vi "fast scanner v1.1.vi"() -> ()   [LabVIEW 2015]
uses:
  outofrange.ctl
  loopclock.ctl
  libs/fast scanner.ctl
  <vilib>/Utility/file.llb/Write Delimited Spreadsheet (I64).vi
  Zaber A Series/Zaber A Series.lvlib
panel:
  in  "Data folder path":path=path "d:/Users/XRF/Desktop/Scan DATA"
  out "DANTE loaded":bool
  out "IP added":bool
  out "Library Initialized":bool
  out "DANTE configured":bool
  out "Enum":T1=enum."MoveToStartPoint"
  out "scan mode":bool
  out "Port":refnum<visa-resource-name>
  out "MotorsReady":bool
  out "Speed 2":T2 scale=0.0..30.0
  in  "Tab Control":T3(tab)
  in  "StopMotion":bool
  in  "GoToZ":bool
  in  "GoToY":bool
  in  "GoToX":bool
  in  "GoTo Z [mm]":dbl format="%#.8g"
  in  "GoTo Y [mm]":dbl format="%#.8g"
  in  "GoTo X [mm]":dbl format="%#.8g"
  in  "Reduced Speed":bool
  in  "Speed Z [mm/s]":dbl(slide) caption="Z Speed\n[mm/s]" min=0.5 max=10.0 step=0.5 scale=0.5..10.0
  in  "XY Speed\n[mm/s]":dbl(slide)=1.0 min=1.0 max=75.0 step=1.0 scale=1.0..75.0
  in  "Away":bool
  in  "Closer":bool
  in  "Right":bool
  in  "Left":bool
  in  "Down":bool
  in  "Up":bool
  out "X [mm]":dbl format="%#.8g"
  out "Y [mm]":dbl format="%#.8g"
  out "Z [mm]":dbl format="%#.3g"
  out "Assignment":cluster{"Microstep Size":dbl, "Device":string}[](array[cluster])
  in  "Acceleration [mm/s^2]":dbl=1.0 min=1.0 max=488.0
  out "SpectraPlot":dbl[](graph) caption="Waveform Graph"
  in  "APPEARANCE_CursorVis":bool
  in  "APPEARANCE_Log/Lin":bool=TRUE
  out "stats out":T4
  out "identifier out":string
  in  "IP Address":string="10.96.0.110"
  out "Progress":u32 caption="%" min=1 step=1
  in  "Preset Time [s]":dbl=1.0 min=0.2 step=0.1
  out "Elapsed Time":dbl caption="Elapsed Time [s]" format="%#_4g"
  in  "MEASUREMENT_Start":bool
  in  "INIT DANTE":bool
  in  "Close DANTE":bool
  out "ROI Begin":u32 caption="ROI begin channel"
  out "ROI End":u32 caption="ROI end channel"
  in  "X velocity [mm/s]":dbl=50.0 min=0.0 step=0.1
  out "Total scan time [s]":dbl=1.0 min=0.0 step=0.1
  out "Total line time [s]":dbl=1.0 min=0.0 step=0.1
  out "Acq time [s]":dbl=1.0 min=0.0 step=0.1
  in  "AcqStartDelay":dbl caption="Acq start delay [ms]"
  in  "Abort scan":bool
  out "Acc time [s]":dbl=1.0 min=0.0 step=0.1
  out "Acc dist [mm]":dbl=1.0 caption="Single line measurement time:" min=0.0 step=0.1
  in  "X accel":dbl caption="X acceleration [mm/s^2]"
  out "Line #":i32=1 caption="/" min=0 step=1
  out "X scan velocity [mm/s]":dbl=1.0 min=0.0 step=0.1
  in  "QUICKSCAN_Start":bool
  out "Y error":T5
  out "X error":T5
  out "total # of points":i32=1 min=0 step=1
  out "Y steps":i32=1 min=1 step=1
  out "X steps":i32=1 min=1 step=1
  in  "step Y [mm]":dbl=1.0 min=0.0 step=0.1
  in  "Y end [mm]":dbl=1.0
  in  "Y start [mm]":dbl
  in  "step X [mm]":dbl=1.0 min=0.0 step=0.1
  in  "X end [mm]":dbl=1.0
  in  "X start [mm]":dbl
  in  "PresetVal":u32 caption="Time per pixel [ms]"
  out "X speed error":T5
  out "total line #":i32=1 caption="/" min=0 step=1
  out "Return movement time [s]":dbl=1.0 min=0.0 step=0.1
  out "ROI map":u32[][](graph)
  out "Sum spectra":u32[](graph)
  out "Spectra":u16[][](graph)
  out "scan timing [ms]":dbl[][](array[numeric])
  out "Y positions array":dbl[](array[numeric])
  out "X start position":dbl
  out "X end position":dbl
  in  "Precision [mm]":dbl=0.1
  out "ZaberError":errorcluster
  out "Loop Speed [1/s]":dbl caption="Elapsed Time [s]" format="%#_2f"
  # "waiting \ntill stage \nreaches \nproper speed"
  # "sending \nmovement \ncommand"
  # "waiting till \nstage stops \n(breaking)"
  # "aquisition"
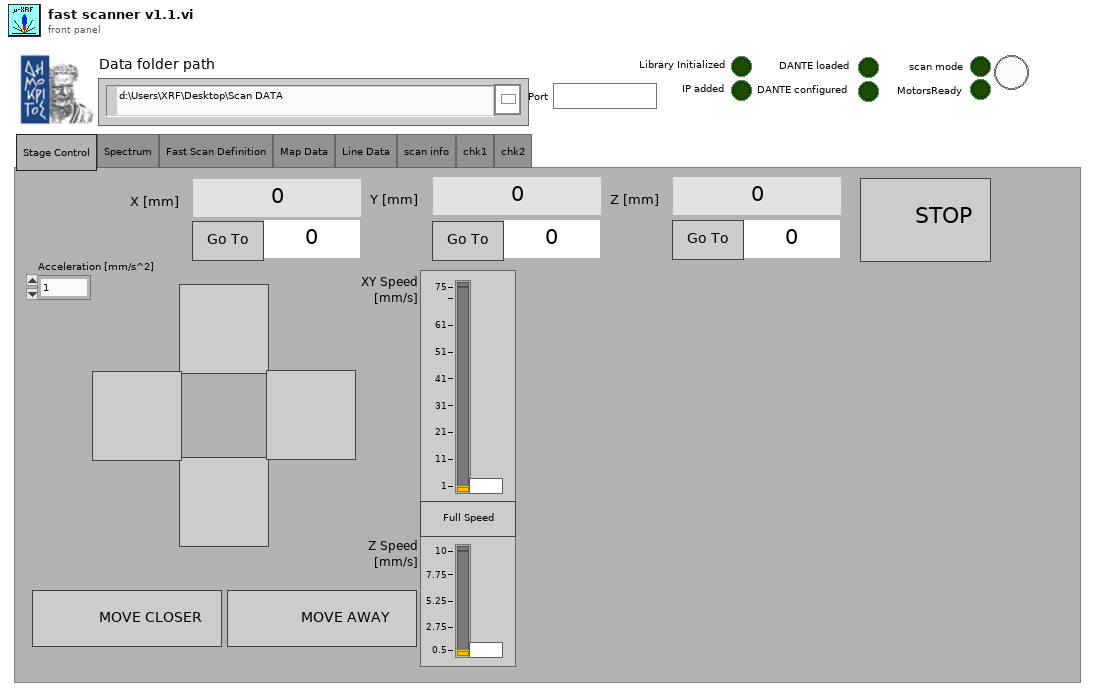
[diagram p1: front panel]
types:
  T1 = typedef "fast scanner.ctl" = enum16{"Initialisation", "IDLE", "Acquire", "PrepareMap", "MoveToStartPoint", "AcquireLine", "Close"}
  T2 = typedef "loopclock.ctl" = dbl
  T3 = enum32{"Stage Control", "Spectrum", "Fast Scan Definition", "Map Data", "Line Data", "scan info", "chk1", "chk2"}
  T4 = cluster{u64, u64, dbl, dbl, u32, u32, u32, u32, u32, u32, u32, u32, u32, u32, u32}
  T5 = typedef "outofrange.ctl" = bool
  T6 = cluster{"X min":dbl, "X max":dbl, "Y min":dbl, "Y max":dbl, "Z min":dbl, "Z max":dbl}
  T7 = enum32{"Size Tabs To Contents", "Size All Tabs to Largest Tab", "Fixed Tab Size"}
  T8 = enum8{"Enabled", "Disabled", "Disabled and Grayed Out"}
  T9 = typedef "LVMinMaxIncTypeDef.ctl" = cluster{"Minimum":dbl, "Maximum":dbl, "Increment":dbl}
  T10 = typedef "LVRangeTypeDef.ctl" = cluster{"Minimum":dbl, "Maximum":dbl, "Increment":dbl, "Minor Increment":dbl, "Start":dbl}
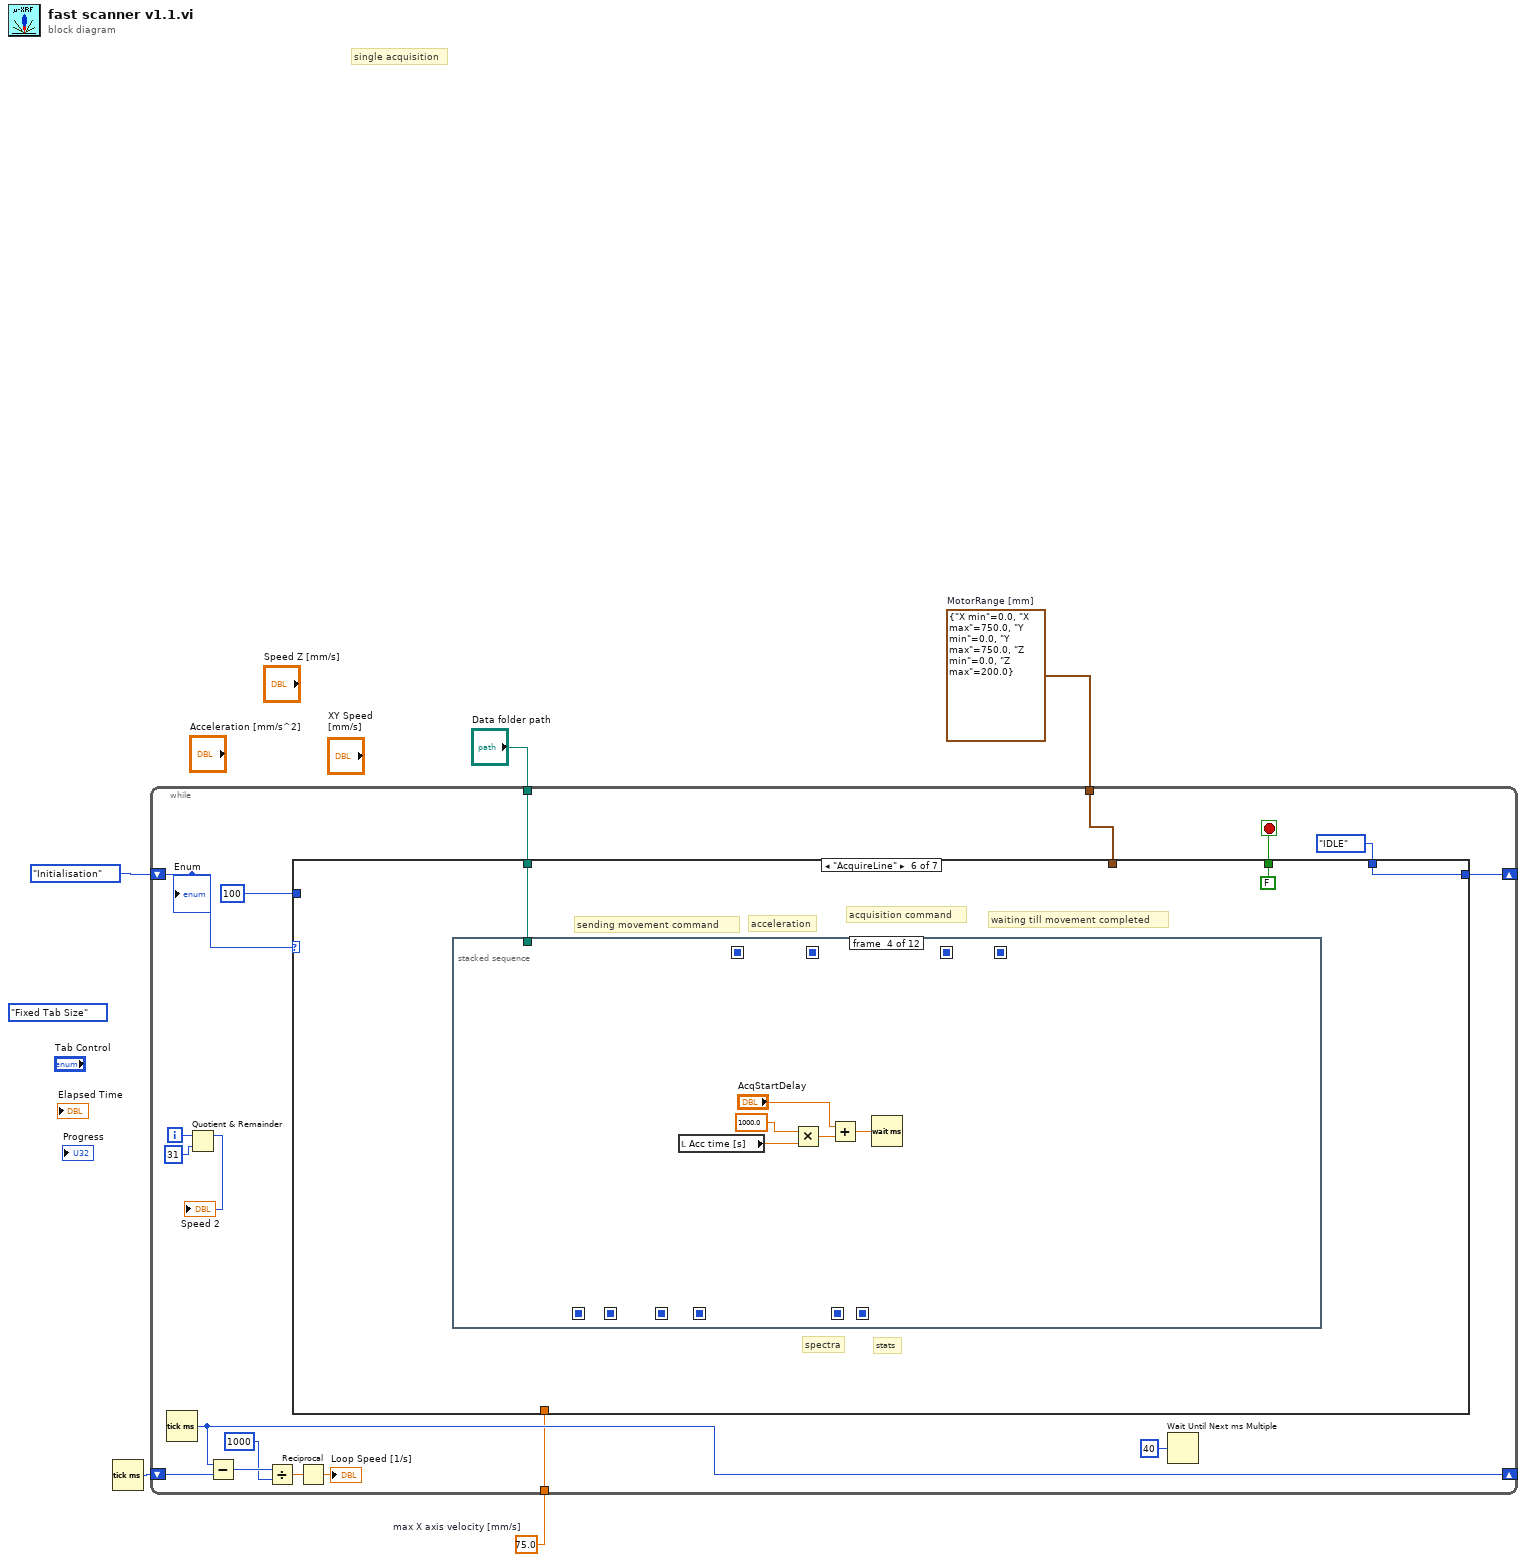
[diagram p0: block diagram]
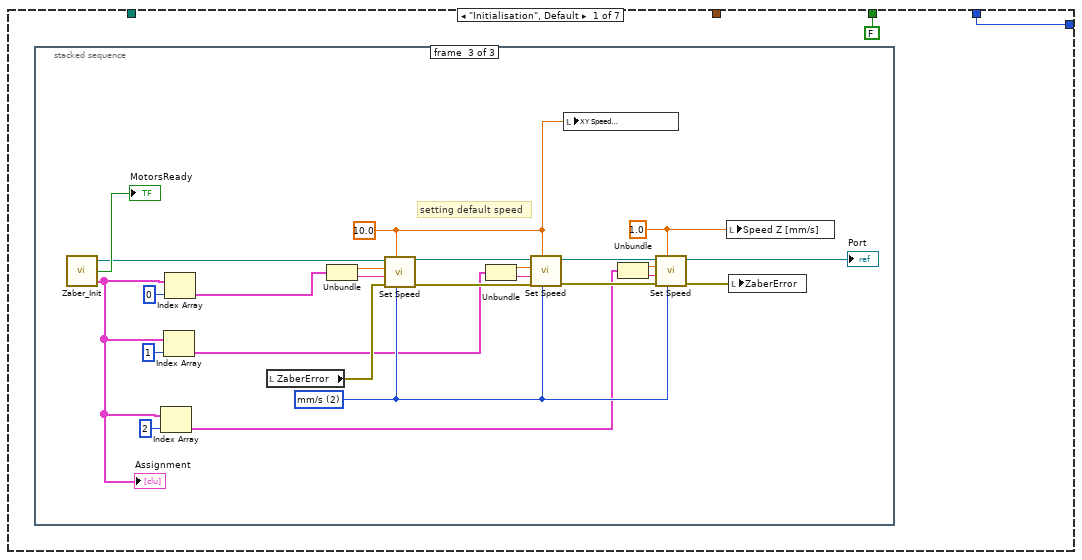
[diagram p2: hidden frame]
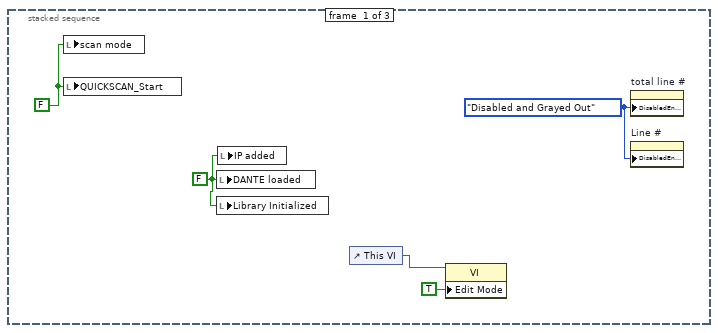
[diagram p3: hidden frame]
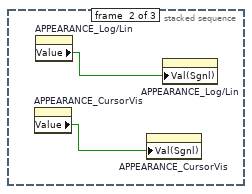
[diagram p4: hidden frame]
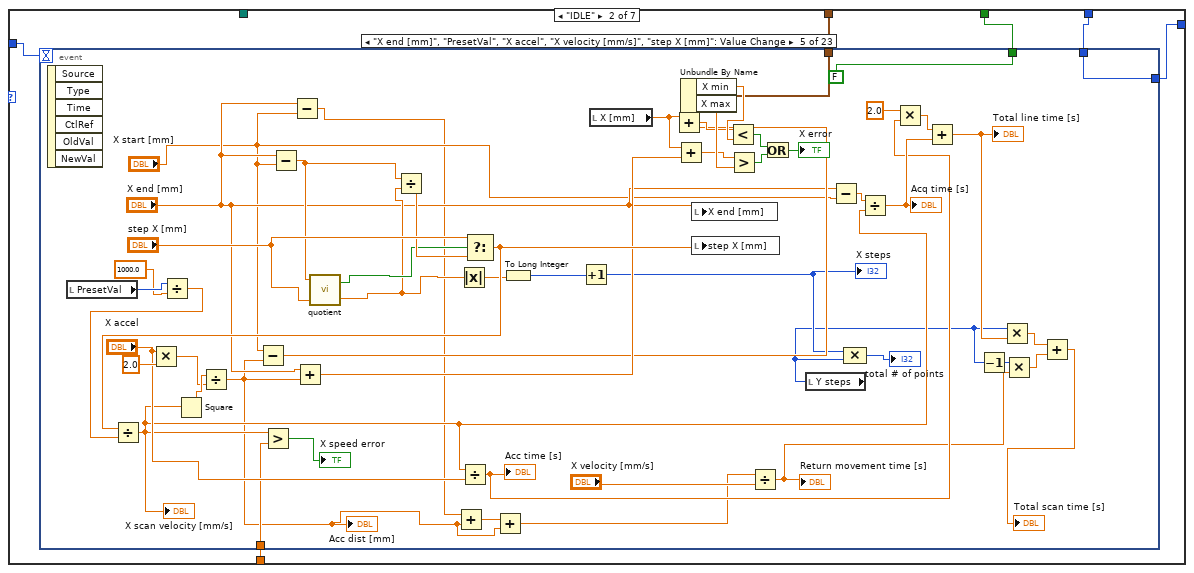
[diagram p5: hidden frame]
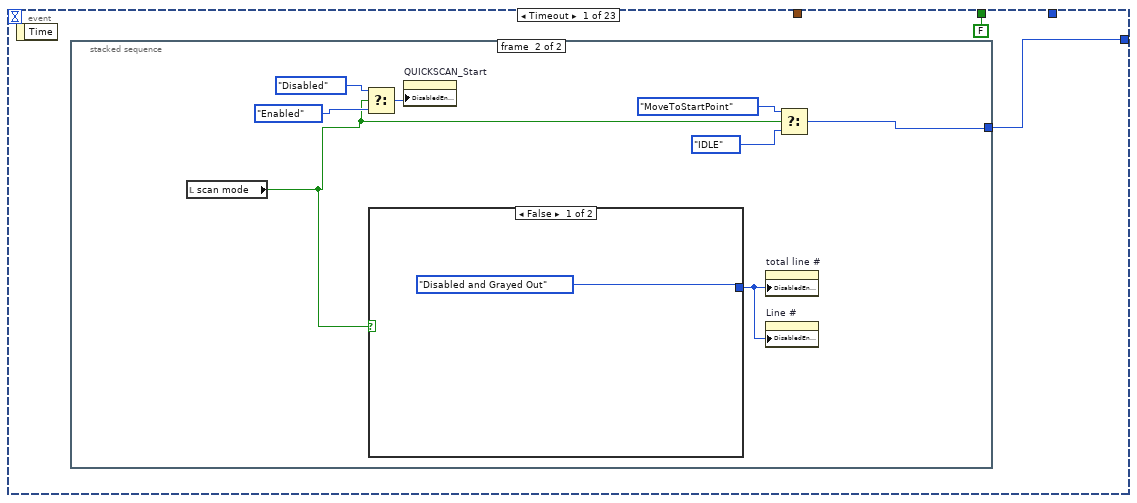
[diagram p6: hidden frame]
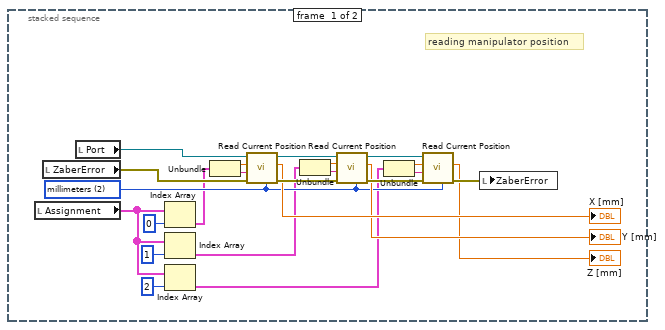
[diagram p7: hidden frame]
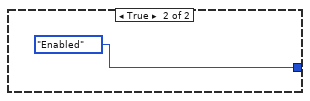
[diagram p8: hidden frame]
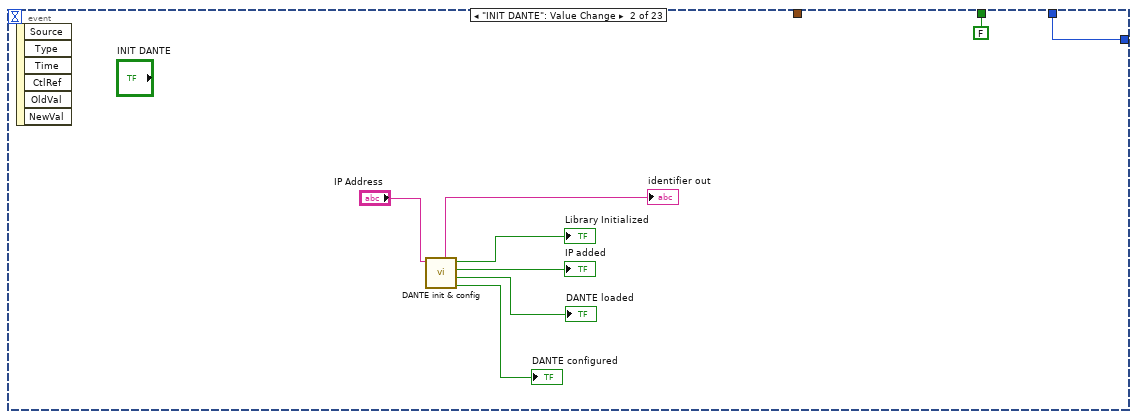
[diagram p9: hidden frame]
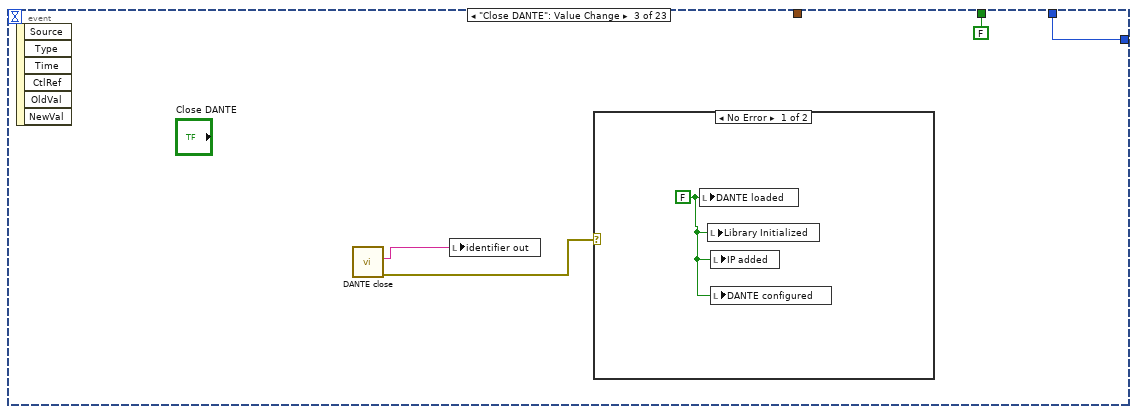
[diagram p10: hidden frame]
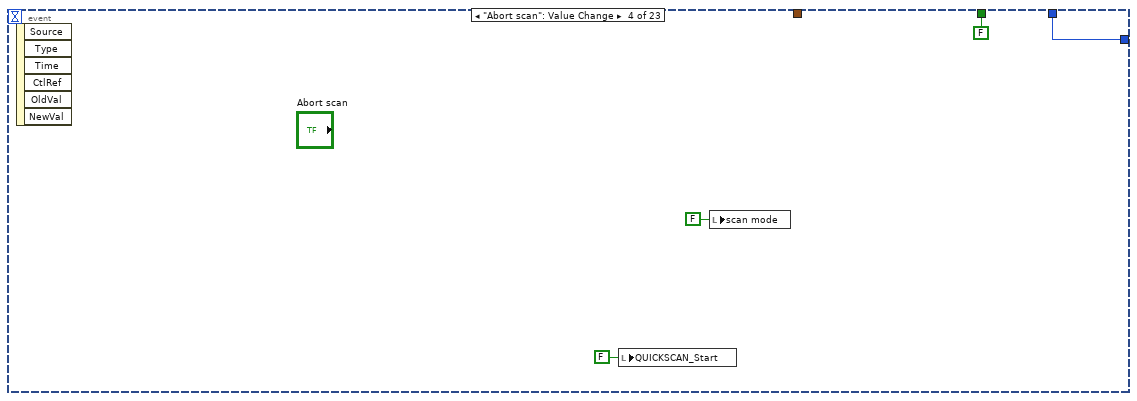
[diagram p12: hidden frame]
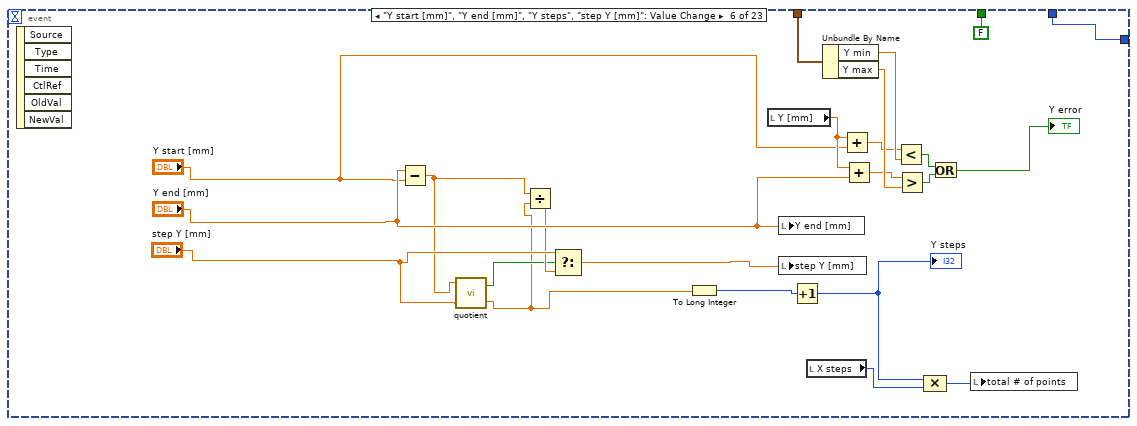
[diagram p13: hidden frame]
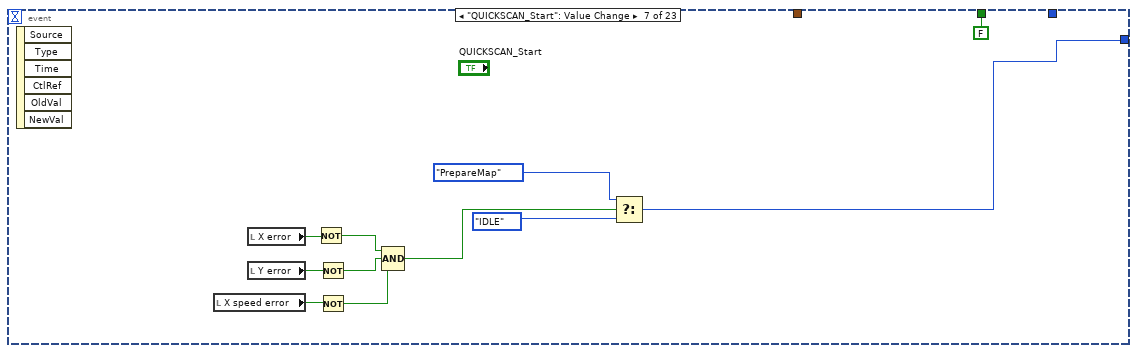
[diagram p14: hidden frame]
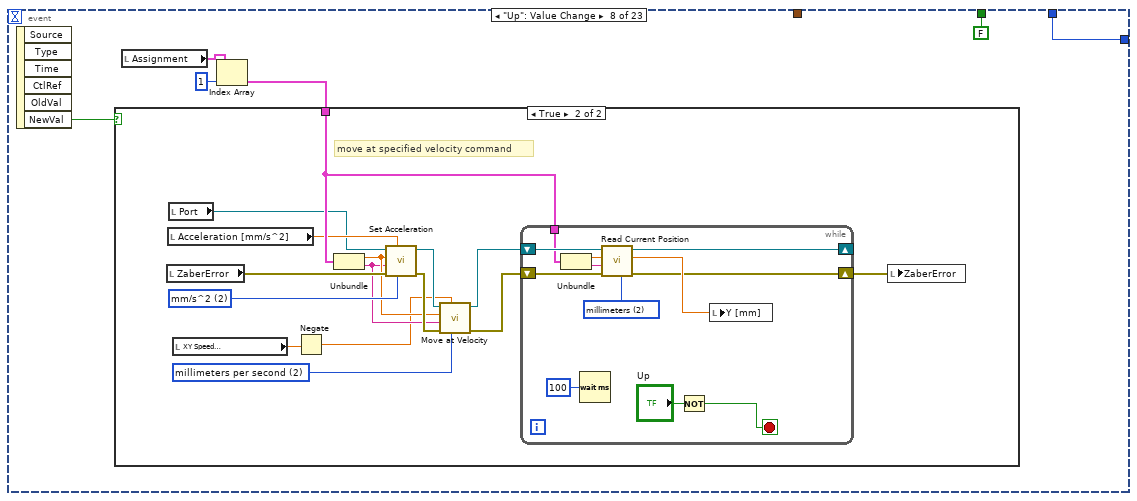
[diagram p15: hidden frame]
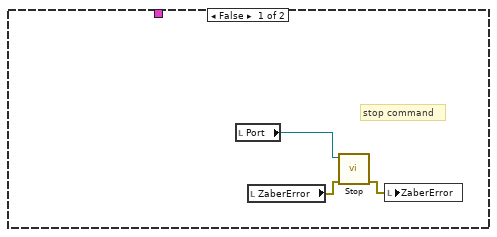
[diagram p16: hidden frame]
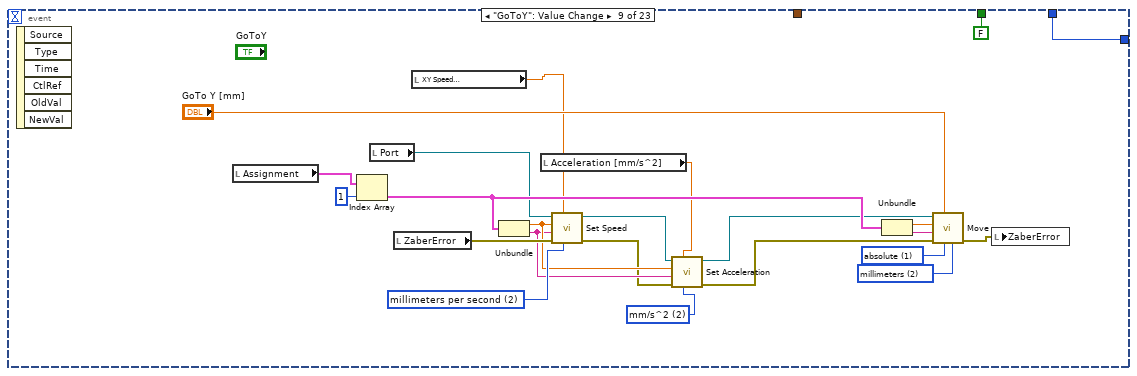
[diagram p17: hidden frame]
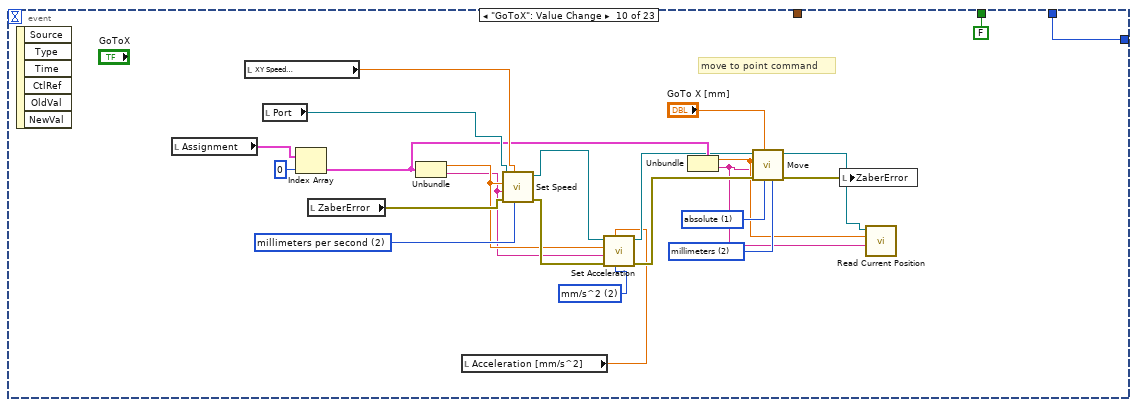
[diagram p18: hidden frame]
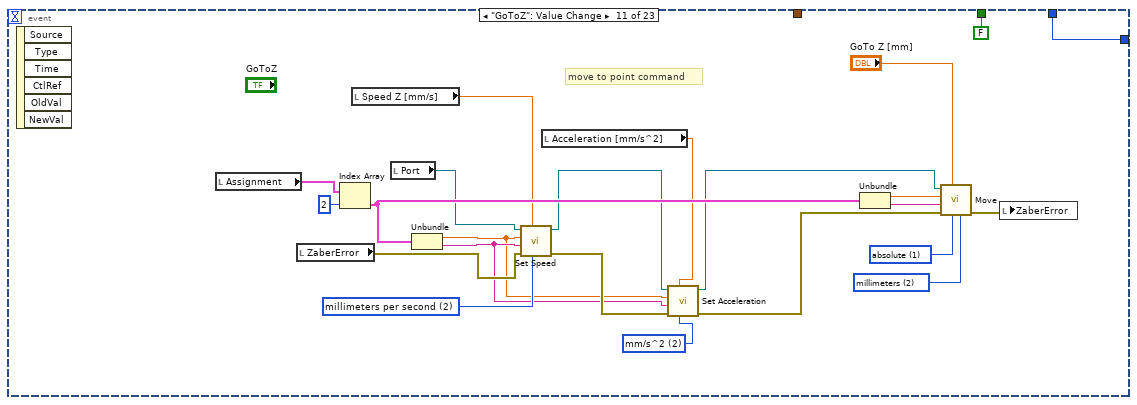
[diagram p19: hidden frame]
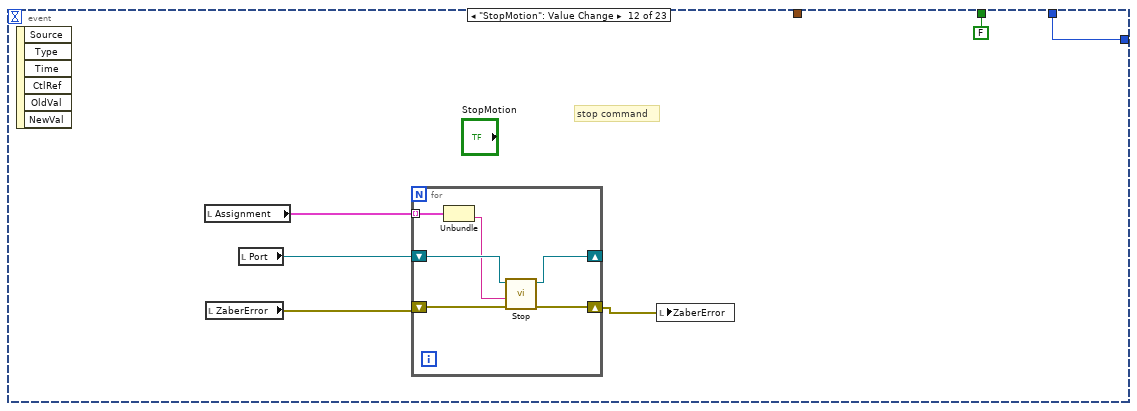
[diagram p20: hidden frame]
diagram:
  w2 = 75.0  # max X axis velocity [mm/s]
  w4 = T6 {"X min"=0.0, "X max"=750.0, "Y min"=0.0, "Y max"=750.0, "Z min"=0.0, "Z max"=200.0}  # MotorRange [mm]
  (unwired) T7."Fixed Tab Size" ("Tab Size")
  # "single acquisition"
  n1 = Tick Count (ms)() -> (millisecond timer value=w5:u32)
  n2 = while {
    shift-right: [w12] -> _
    shift-left: fast_scanner."Initialisation" ("Enum") -> [w8]
    shift-right: [w19] -> _
    shift-left: w5 -> [w23]
    tunnel: w4 -> [w9]
    tunnel: w2 -> [w7]
    tunnel: "Data folder path" -> [w6]
    i -> [w18]
    stop <- w11 stop-if-true
    n3 = Tick Count (ms)() -> (millisecond timer value=w19:u32)
    n4 = Quotient & Remainder(x=w18, y=31) -> (x-y*floor(x/y)=→"Speed 2":i32)  [unwired: 1 out]
    n5 = Subtract(x=w19, y=w23) -> (x-y=w21:u32)
    n6 = Divide(x=w21, y=u32 1000) -> (x/y=w22:dbl)
    n7 = case shown="\"AcquireLine\"" w8 {
      tunnel: 100 ("LoopTimer [ms]") -> [_ w59 _ _ _ _ _]
      tunnel: [w25 w61 fast_scanner."IDLE" ("Enum") w573 fast_scanner."AcquireLine" ("Enum") w683 fast_scanner."Close" ("Enum")] -> w12
      tunnel: [FALSE ("VI stop") w60 FALSE ("VI stop") FALSE ("VI stop") FALSE ("VI stop") FALSE ("VI stop") TRUE ("VI stop")] -> w11
      tunnel: fast_scanner."IDLE" ("Enum") -> [w25 w63 _ w573 _ w683 _]
      tunnel: w9 -> [_ w62 _ _ _ _ _]
      tunnel: w7 -> [_ w58 _ _ _ _ _]
      tunnel: w6 -> [_ _ _ _ _ w682 _]
      frame "Initialisation", Default {
        n8 = stacked-sequence {
          frame #0 {
            w26 = FALSE ("DANTE loaded")
            w27 = T8."Disabled and Grayed Out" ("Disabled")
            w28 = FALSE ("batch mode")
            n9 = local write "scan mode"(w28) -> ()
            n10 = local write "QUICKSCAN_Start"(w28) -> ()
            n11 = local write "DANTE loaded"(w26) -> ()
            n12 = local write "Library Initialized"(w26) -> ()
            n13 = local write "IP added"(w26) -> ()
            n14 = control-ref of="This VI"() -> (w29:refnum<vi>)
            n15 = property class="VI"(reference=w29, "Edit Mode"=TRUE ("Edit Mode On Open")) -> ()  [unwired: 1 in, 2 out]
            n16 = property on="total line #" class="DigNum (strict)"("DisabledEnum"=w27) -> ()  [unwired: 2 in, 2 out]
            n17 = property on="Line #" class="DigNum (strict)"("DisabledEnum"=w27) -> ()  [unwired: 2 in, 2 out]
          }
          frame #1 {
            n18 = property on="APPEARANCE_CursorVis" class="Bool (strict)"() -> ("Value"=w31:bool)  [unwired: 2 in, 2 out]
            n19 = property on="APPEARANCE_Log/Lin" class="Bool (strict)"() -> ("Value"=w32:bool)  [unwired: 2 in, 2 out]
            n20 = property on="APPEARANCE_CursorVis" class="Bool (strict)"("Val(Sgnl)"=w31) -> ()  [unwired: 2 in, 2 out]
            n21 = property on="APPEARANCE_Log/Lin" class="Bool (strict)"("Val(Sgnl)"=w32) -> ()  [unwired: 2 in, 2 out]
          }
          frame #2 {
            w42 = 1.0 ("New Speed")
            w43 = 10.0 ("New Speed")
            w46 = u16 2 items=["device units", "microns/s", "mm/s", "inches/s", "degrees/s"] ("Units (0: data)")
            # "setting default speed"
            n22 = call "Zaber_Init.vi"() -> ("Assignment"=w47:cluster{"Microstep Size":dbl, "Device":string}[], "Axes Ass"=→"MotorsReady":bool, "VISA resource name out"=w55:refnum<visa-resource-name>)
            "Assignment" <- w47
            n23 = Index Array(array=w47, index=2) -> (element=w34:cluster{"Microstep Size":dbl, "Device":string})
            n24 = Index Array(array=w47, index=1) -> (element=w36:cluster{"Microstep Size":dbl, "Device":string})
            n25 = Index Array(array=w47, index=0) -> (element=w41:cluster{"Microstep Size":dbl, "Device":string})
            n26 = local read "ZaberError"() -> (w56:errorcluster)
            n27 = Unbundle(w41) -> ("Microstep Size"=w40:dbl, "Device"=w39:string)
            n28 = call "Set Speed.vi"("Units (0: data)"=w46, "New Speed"=w43, "error in (no error)"=w56, "Device and Axis"=w39, "Microstep Size (0)"=w40, "VISA resource name"=w55) -> ("error out"=w52:errorcluster, "VISA resource name out"=w51:refnum<visa-resource-name>)  [unwired: 4 in]
            n29 = Unbundle(w36) -> ("Microstep Size"=w37:dbl, "Device"=w38:string)
            n30 = call "Set Speed.vi"("Units (0: data)"=w46, "New Speed"=w43, "error in (no error)"=w52, "Device and Axis"=w38, "Microstep Size (0)"=w37, "VISA resource name"=w51) -> ("error out"=w49:errorcluster, "VISA resource name out"=w50:refnum<visa-resource-name>)  [unwired: 4 in]
            n31 = local write "XY Speed\n[mm/s]"(w43) -> ()
            n32 = Unbundle(w34) -> ("Microstep Size"=w35:dbl, "Device"=w33:string)
            n33 = call "Set Speed.vi"("Units (0: data)"=w46, "New Speed"=w42, "error in (no error)"=w49, "Device and Axis"=w33, "Microstep Size (0)"=w35, "VISA resource name"=w50) -> ("error out"=w45:errorcluster, "VISA resource name out"=→"Port":refnum<visa-resource-name>)  [unwired: 4 in]
            n34 = local write "Speed Z [mm/s]"(w42) -> ()
            n35 = local write "ZaberError"(w45) -> ()
          }
        }
      }
      frame "IDLE" {
        n36 = event shown="[4] \"X end [mm]\", \"PresetVal\", \"X accel\", \"X velocity [mm/s]\", \"step X [mm]\": Value Change" {
          selector: _ -> [_ _ _ _ _ _ _ _ _ _ _ _ _ _ _ _ _ _ _ _ _ _ _]
          dyn-events: _ -> [_ _ _ _ _ _ _ _ _ _ _ _ _ _ _ _ _ _ _ _ _ _ _]
          timeout: w59 -> [_ _ _ _ _ _ _ _ _ _ _ _ _ _ _ _ _ _ _ _ _ _ _]
          tunnel: [FALSE ("VI stop") FALSE ("VI stop") FALSE ("VI stop") FALSE ("VI stop") FALSE ("VI stop") FALSE ("VI stop") FALSE ("VI stop") FALSE ("VI stop") FALSE ("VI stop") FALSE ("VI stop") FALSE ("VI stop") FALSE ("VI stop") FALSE ("VI stop") FALSE ("VI stop") FALSE ("VI stop") FALSE ("VI stop") FALSE ("VI stop") FALSE ("VI stop") TRUE ("VI stop") FALSE ("VI stop") FALSE ("VI stop") FALSE ("VI stop") FALSE ("VI stop")] -> w60
          tunnel: [w64 w107 w111 w115 w168 w189 w192 w206 w260 w284 w307 w314 w325 w360 w395 w431 w466 w510 w527 fast_scanner."Acquire" ("Enum") w545 w550 w554] -> w61
          tunnel: w63 -> [_ w107 w111 w115 w168 w189 _ w206 w260 w284 w307 w314 w325 w360 w395 w431 w466 w510 _ _ w545 w550 w554]
          tunnel: w62 -> [_ _ _ _ w156 w175 _ _ _ _ _ _ _ _ _ _ _ _ _ _ _ _ _]
          tunnel: w58 -> [_ _ _ _ w145 _ _ _ _ _ _ _ _ _ _ _ _ _ _ _ _ _ _]
          event Timeout {
            n37 = event-data() -> ()  [unwired: 1 in, 1 out]
            n38 = stacked-sequence {
              tunnel: [_ w97] -> w64
              frame #0 {
                w76 = u16 2 items=["microsteps", "microns", "millimeters", "inches"] ("Units (0: microsteps)")
                # "reading manipulator position"
                n39 = local read "Assignment"() -> (w75:cluster{"Microstep Size":dbl, "Device":string}[])
                n40 = local read "ZaberError"() -> (w88:errorcluster)
                n41 = local read "Port"() -> (w89:refnum<visa-resource-name>)
                n42 = Index Array(array=w75, index=0) -> (element=w74:cluster{"Microstep Size":dbl, "Device":string})
                n43 = Index Array(array=w75, index=1) -> (element=w70:cluster{"Microstep Size":dbl, "Device":string})
                n44 = Index Array(array=w75, index=2) -> (element=w66:cluster{"Microstep Size":dbl, "Device":string})
                n45 = Unbundle(w74) -> ("Microstep Size"=w73:dbl, "Device"=w72:string)
                n46 = call "Read Current Position.vi"("Units (0: microsteps)"=w76, "error in (no error)"=w88, "Device and Axis"=w72, "Microstep Size (0)"=w73, "VISA resource name"=w89) -> ("error out"=w87:errorcluster, "Position"=→"X [mm]":dbl, "VISA resource name out"=w86:refnum<visa-resource-name>)  [unwired: 4 in]
                n47 = Unbundle(w70) -> ("Microstep Size"=w71:dbl, "Device"=w69:string)
                n48 = call "Read Current Position.vi"("Units (0: microsteps)"=w76, "error in (no error)"=w87, "Device and Axis"=w69, "Microstep Size (0)"=w71, "VISA resource name"=w86) -> ("error out"=w85:errorcluster, "Position"=→"Y [mm]":dbl, "VISA resource name out"=w84:refnum<visa-resource-name>)  [unwired: 4 in]
                n49 = Unbundle(w66) -> ("Microstep Size"=w68:dbl, "Device"=w67:string)
                n50 = call "Read Current Position.vi"("Units (0: microsteps)"=w76, "error in (no error)"=w85, "Device and Axis"=w67, "Microstep Size (0)"=w68, "VISA resource name"=w84) -> ("error out"=w83:errorcluster, "Position"=→"Z [mm]":dbl)  [unwired: 4 in, 1 out]
                n51 = local write "ZaberError"(w83) -> ()
              }
              frame #1 {
                n52 = local read "scan mode"() -> (w90:bool)
                n53 = Select(t=T8."Disabled" ("Disabled"), s=w90, f=T8."Enabled" ("Disabled")) -> (s? t:f=w94:T8)
                n54 = case shown="False" w90 {
                  tunnel: [T8."Disabled and Grayed Out" ("Disabled") T8."Enabled" ("Disabled")] -> w91
                  frame False {
                  }
                  frame True {
                  }
                }
                n55 = property on="QUICKSCAN_Start" class="Bool (strict)"("DisabledEnum"=w94) -> ()  [unwired: 2 in, 2 out]
                n56 = property on="total line #" class="DigNum (strict)"("DisabledEnum"=w91) -> ()  [unwired: 2 in, 2 out]
                n57 = property on="Line #" class="DigNum (strict)"("DisabledEnum"=w91) -> ()  [unwired: 2 in, 2 out]
                n58 = Select(t=fast_scanner."MoveToStartPoint" ("Enum"), s=w90, f=fast_scanner."IDLE" ("Enum")) -> (s? t:f=w97:T1)
              }
            }
          }
          event "INIT DANTE": Value Change {
            n59 = event-data() -> ()  [unwired: 1 in, 6 out]
            n60 = call "DANTE init & config.vi"("IP Address"="IP Address") -> ("DANTE configured"=→"DANTE configured":bool, "DANTE loaded"=→"DANTE loaded":bool, "IP added"=→"IP added":bool, "Library Initialized"=→"Library Initialized":bool, "identifier out"=→"identifier out":string)  [unwired: 6 in]
          }
          event "Close DANTE": Value Change {
            n61 = event-data() -> ()  [unwired: 1 in, 6 out]
            n62 = call "DANTE close.vi"() -> ("error out"=w108:errorcluster, "identifier out"=w109:string)  [unwired: 9 in, 1 out]
            n63 = local write "identifier out"(w109) -> ()
            n64 = case shown="No Error" w108 {
              frame No Error {
                w112 = FALSE ("DANTE loaded")
                n65 = local write "DANTE loaded"(w112) -> ()
                n66 = local write "Library Initialized"(w112) -> ()
                n67 = local write "IP added"(w112) -> ()
                n68 = local write "DANTE configured"(w112) -> ()
              }
              frame Error {
              }
            }
          }
          event "Abort scan": Value Change {
            n69 = event-data() -> ()  [unwired: 1 in, 6 out]
            n70 = local write "QUICKSCAN_Start"(FALSE ("QUICKSCAN_Start")) -> ()
            n71 = local write "scan mode"(FALSE ("scan mode")) -> ()
          }
          event "X end [mm]", "PresetVal", "X accel", "X velocity [mm/s]", "step X [mm]": Value Change {
            n72 = event-data() -> ()  [unwired: 1 in, 6 out]
            n73 = local read "PresetVal"() -> (w152:u32)
            n74 = Multiply(x="X accel", y=2.0) -> (x*y=w147:dbl)
            n75 = Divide(x=w152, y=1000.0 ("x")) -> (x/y=w150:dbl)
            n76 = Subtract(x="X end [mm]", y="X start [mm]") -> (x-y=w139:dbl)
            n77 = Subtract(x="X end [mm]", y="X start [mm]") -> (x-y=w120:dbl)
            n78 = call "quotient.vi"("Y"="step X [mm]", "X"=w139) -> ("s? t:f"=w137:dbl, "x = y?"=w138:bool)  [unwired: 1 in]
            n79 = Divide(x=w139, y=w137) -> (x/y=w141:dbl)
            n80 = Absolute Value(x=w137) -> (abs(x)=w140:dbl)
            n81 = Select(t="step X [mm]", s=w138, f=w141) -> (s? t:f=w154:dbl)
            n82 = Divide(x=w154, y=w150) -> (x/y=w134:dbl)
            "X scan velocity [mm/s]" <- w134
            n83 = Square(x=w134) -> (x^2=w149:dbl)
            n84 = Divide(x=w149, y=w147) -> (x/y=w118:dbl)
            "Acc dist [mm]" <- w118
            n85 = Subtract(x="X start [mm]", y=w118) -> (x-y=w143:dbl)
            n86 = Greater?(x=w134, y=w145) -> (0:→"X speed error":bool)
            n87 = Add(x="X end [mm]", y=w118) -> (x+y=w144:dbl)
            n88 = Add(x=w120, y=w118) -> (x+y=w119:dbl)
            n89 = Divide(x=w134, y="X accel") -> (x/y=w130:dbl)
            "Acc time [s]" <- w130
            n90 = Add(x=w119, y=w118) -> (x+y=w117:dbl)
            n91 = To Long Integer(number=w140) -> (32bit integer=w160:i32)
            n92 = Increment(x=w160) -> (x+1=w136:i32)
            "X steps" <- w136
            n93 = local read "X [mm]"() -> (w164:dbl)
            n94 = Add(x=w164, y=w143) -> (x+y=w159:dbl)
            n95 = Add(x=w164, y=w144) -> (x+y=w158:dbl)
            n96 = Unbundle By Name(w156) -> ("X min"=w165:dbl, "X max"=w163:dbl)
            n97 = local write "X end [mm]"("X end [mm]") -> ()
            n98 = local write "step X [mm]"(w154) -> ()
            n99 = Less?(x=w159, y=w165) -> (x < y?=w161:bool)
            n100 = Greater?(x=w158, y=w163) -> (0:w162:bool)
            n101 = Divide(x=w117, y="X velocity [mm/s]") -> (x/y=w126:dbl)
            "Return movement time [s]" <- w126
            n102 = Or(x=w161, y=w162) -> (x .or. y?=→"X error":bool)
            n103 = local read "Y steps"() -> (w127:i32)
            n104 = Subtract(x="X end [mm]", y="X start [mm]") -> (x-y=w135:dbl)
            n105 = Compound Arithmetic op=MULTIPLY(w136, w127) -> (→"total # of points":i32)
            n106 = Divide(x=w135, y=w134) -> (x/y=w133:dbl)
            "Acq time [s]" <- w133
            n107 = Multiply(x=2.0, y=w130) -> (x*y=w132:dbl)
            n108 = Add(x=w132, y=w133) -> (x+y=w129:dbl)
            "Total line time [s]" <- w129
            n109 = Decrement(x=w127) -> (x-1=w128:i32)
            n110 = Multiply(x=w127, y=w129) -> (x*y=w124:dbl)
            n111 = Multiply(x=w128, y=w126) -> (x*y=w125:dbl)
            n112 = Add(x=w124, y=w125) -> (x+y=→"Total scan time [s]":dbl)
          }
          event "Y start [mm]", "Y end [mm]", "Y steps", "step Y [mm]": Value Change {
            n113 = event-data() -> ()  [unwired: 1 in, 6 out]
            n114 = Subtract(x="Y end [mm]", y="Y start [mm]") -> (x-y=w172:dbl)
            n115 = call "quotient.vi"("Y"="step Y [mm]", "X"=w172) -> ("s? t:f"=w170:dbl, "x = y?"=w171:bool)  [unwired: 1 in]
            n116 = Divide(x=w172, y=w170) -> (x/y=w173:dbl)
            n117 = Select(t="step Y [mm]", s=w171, f=w173) -> (s? t:f=w176:dbl)
            n118 = To Long Integer(number=w170) -> (32bit integer=w187:i32)
            n119 = local read "Y [mm]"() -> (w185:dbl)
            n120 = local write "Y end [mm]"("Y end [mm]") -> ()
            n121 = local write "step Y [mm]"(w176) -> ()
            n122 = Increment(x=w187) -> (x+1=w169:i32)
            "Y steps" <- w169
            n123 = local read "X steps"() -> (w186:i32)
            n124 = Unbundle By Name(w175) -> ("Y min"=w181:dbl, "Y max"=w180:dbl)
            n125 = Add(x=w185, y="Y start [mm]") -> (x+y=w178:dbl)
            n126 = Add(x=w185, y="Y end [mm]") -> (x+y=w177:dbl)
            n127 = Less?(x=w178, y=w181) -> (x < y?=w183:bool)
            n128 = Greater?(x=w177, y=w180) -> (0:w184:bool)
            n129 = Compound Arithmetic op=MULTIPLY(w169, w186) -> (w174:i32)
            n130 = Or(x=w183, y=w184) -> (x .or. y?=→"Y error":bool)
            n131 = local write "total # of points"(w174) -> ()
          }
          event "QUICKSCAN_Start": Value Change {
            n132 = event-data() -> ()  [unwired: 1 in, 6 out]
            n133 = local read "X speed error"() -> (w198:T5)
            n134 = local read "X error"() -> (w196:T5)
            n135 = local read "Y error"() -> (w197:T5)
            n136 = Not(x=w196) -> (.not. x?=w199:T5)
            n137 = Not(x=w197) -> (.not. x?=w200:T5)
            n138 = Not(x=w198) -> (.not. x?=w201:T5)
            n139 = Compound Arithmetic op=AND(w199, w200, w201) -> (w195:T5)
            n140 = Select(t=fast_scanner."PrepareMap" ("Enum"), s=w195, f=fast_scanner."IDLE" ("Enum")) -> (s? t:f=w192:T1)
          }
          event "Up": Value Change {
            n141 = event-data() -> ("NewVal"=w208:bool)  [unwired: 1 in, 5 out]
            n142 = local read "Assignment"() -> (w203:cluster{"Microstep Size":dbl, "Device":string}[])
            n143 = Index Array(array=w203, index=1) -> (element=w204:cluster{"Microstep Size":dbl, "Device":string})
            n144 = case shown="True" w208 {
              tunnel: w204 -> [_ w225]
              frame False {
                # "stop command"
                n145 = local read "Port"() -> (w211:refnum<visa-resource-name>)
                n146 = local read "ZaberError"() -> (w210:errorcluster)
                n147 = call "Stop.vi"("error in (no error)"=w210, "VISA resource name"=w211) -> ("error out"=w209:errorcluster)  [unwired: 8 in, 1 out]
                n148 = local write "ZaberError"(w209) -> ()
              }
              frame True {
                w223 = u16 2 items=["device units", "microns/s^2", "mm/s^2", "inches/s^2", "degrees/s^2"] ("Units (0: data)")
                w213 = u16 2 items=["device speed units", "microns per second", "millimeters per second", "inches per second", "degrees per second"] ("Units (0: device speed units)")
                # "move at specified velocity command"
                n149 = local read "ZaberError"() -> (w221:errorcluster)
                n150 = local read "Acceleration [mm/s^2]"() -> (w222:dbl)
                n151 = local read "Port"() -> (w220:refnum<visa-resource-name>)
                n152 = local read "XY Speed\n[mm/s]"() -> (w224:dbl)
                n153 = Negate(x=w224) -> (-x=w212:dbl)
                n154 = Unbundle(w225) -> ("Microstep Size"=w217:dbl, "Device"=w216:string)
                n155 = call "Set Acceleration.vi"("Units (0: data)"=w223, "New Acceleration"=w222, "error in (no error)"=w221, "Device and Axis"=w216, "Microstep Size (0)"=w217, "VISA resource name"=w220) -> ("error out"=w219:errorcluster, "VISA resource name out"=w218:refnum<visa-resource-name>)  [unwired: 4 in]
                n156 = call "Move at Velocity.vi"("Units (0: device speed units)"=w213, "Velocity"=w212, "error in (no error)"=w219, "Device and Axis"=w216, "Microstep Size (0)"=w217, "VISA resource name"=w218) -> ("error out"=w214:errorcluster, "VISA resource name out"=w215:refnum<visa-resource-name>)  [unwired: 4 in]
                n157 = while {
                  shift-right: [w230] -> _
                  shift-left: w215 -> [w233]
                  shift-right: [w231] -> w226
                  shift-left: w214 -> [w232]
                  tunnel: w225 -> [w229]
                  stop <- w236 stop-if-true
                  w235 = u16 2 items=["microsteps", "microns", "millimeters", "inches"] ("Units (0: microsteps)")
                  n158 = Unbundle(w229) -> ("Microstep Size"=w228:dbl, "Device"=w227:string)
                  n159 = Wait (ms)(milliseconds to wait=u32 100) -> ()  [unwired: 1 out]
                  n160 = call "Read Current Position.vi"("Units (0: microsteps)"=w235, "error in (no error)"=w232, "Device and Axis"=w227, "Microstep Size (0)"=w228, "VISA resource name"=w233) -> ("error out"=w231:errorcluster, "Position"=w234:dbl, "VISA resource name out"=w230:refnum<visa-resource-name>)  [unwired: 4 in]
                  n161 = Not(x="Up") -> (.not. x?=w236:bool)
                  n162 = local write "Y [mm]"(w234) -> ()
                }
                n163 = local write "ZaberError"(w226) -> ()
              }
            }
          }
          event "GoToY": Value Change {
            w240 = u16 2 items=["device units", "microns/s^2", "mm/s^2", "inches/s^2", "degrees/s^2"] ("Units (0: data)")
            w249 = u16 2 items=["device speed units", "microns per second", "millimeters per second", "inches per second", "degrees per second"] ("Units (0: device speed units)")
            w255 = u16 2 items=["microsteps", "microns", "millimeters", "inches", "degrees"] ("Units (0: microsteps)")
            w258 = u16 1 items=["relative", "absolute"] ("Movement Type (0: relative)")
            n164 = event-data() -> ()  [unwired: 1 in, 6 out]
            n165 = local read "Assignment"() -> (w254:cluster{"Microstep Size":dbl, "Device":string}[])
            n166 = Index Array(array=w254, index=1) -> (element=w251:cluster{"Microstep Size":dbl, "Device":string})
            n167 = local read "Port"() -> (w247:refnum<visa-resource-name>)
            n168 = local read "ZaberError"() -> (w250:errorcluster)
            n169 = local read "XY Speed\n[mm/s]"() -> (w248:dbl)
            n170 = Unbundle(w251) -> ("Microstep Size"=w246:dbl, "Device"=w245:string)
            n171 = local read "Acceleration [mm/s^2]"() -> (w239:dbl)
            n172 = call "Set Speed.vi"("Units (0: data)"=w249, "New Speed"=w248, "error in (no error)"=w250, "Device and Axis"=w245, "Microstep Size (0)"=w246, "VISA resource name"=w247) -> ("error out"=w244:errorcluster, "VISA resource name out"=w242:refnum<visa-resource-name>)  [unwired: 4 in]
            n173 = call "Set Acceleration.vi"("Units (0: data)"=w240, "New Acceleration"=w239, "error in (no error)"=w244, "Device and Axis"=w245, "Microstep Size (0)"=w246, "VISA resource name"=w242) -> ("error out"=w243:errorcluster, "VISA resource name out"=w241:refnum<visa-resource-name>)  [unwired: 4 in]
            n174 = Unbundle(w251) -> ("Microstep Size"=w253:dbl, "Device"=w252:string)
            n175 = call "Move.vi"("Units (0: microsteps)"=w255, "Movement Type (0: relative)"=w258, "Move Distance (0)"="GoTo Y [mm]", "error in (no error)"=w243, "Device and Axis"=w252, "Microstep Size (0)"=w253, "VISA resource name"=w241) -> ("error out"=w256:errorcluster)  [unwired: 3 in, 1 out]
            n176 = local write "ZaberError"(w256) -> ()
          }
          event "GoToX": Value Change {
            w266 = u16 2 items=["device units", "microns/s^2", "mm/s^2", "inches/s^2", "degrees/s^2"] ("Units (0: data)")
            w275 = u16 2 items=["device speed units", "microns per second", "millimeters per second", "inches per second", "degrees per second"] ("Units (0: device speed units)")
            w279 = u16 2 items=["microsteps", "microns", "millimeters", "inches", "degrees"] ("Units (0: microsteps)")
            w281 = u16 1 items=["relative", "absolute"] ("Movement Type (0: relative)")
            # "move to point command"
            n177 = event-data() -> ()  [unwired: 1 in, 6 out]
            n178 = local read "Assignment"() -> (w274:cluster{"Microstep Size":dbl, "Device":string}[])
            n179 = local read "XY Speed\n[mm/s]"() -> (w277:dbl)
            n180 = local read "Port"() -> (w276:refnum<visa-resource-name>)
            n181 = Index Array(array=w274, index=0) -> (element=w273:cluster{"Microstep Size":dbl, "Device":string})
            n182 = local read "ZaberError"() -> (w278:errorcluster)
            n183 = Unbundle(w273) -> ("Microstep Size"=w268:dbl, "Device"=w267:string)
            n184 = local read "Acceleration [mm/s^2]"() -> (w265:dbl)
            n185 = call "Set Speed.vi"("Units (0: data)"=w275, "New Speed"=w277, "error in (no error)"=w278, "Device and Axis"=w267, "Microstep Size (0)"=w268, "VISA resource name"=w276) -> ("error out"=w270:errorcluster, "VISA resource name out"=w272:refnum<visa-resource-name>)  [unwired: 4 in]
            n186 = call "Set Acceleration.vi"("Units (0: data)"=w266, "New Acceleration"=w265, "error in (no error)"=w270, "Device and Axis"=w267, "Microstep Size (0)"=w268, "VISA resource name"=w272) -> ("error out"=w269:errorcluster, "VISA resource name out"=w271:refnum<visa-resource-name>)  [unwired: 4 in]
            n187 = Unbundle(w273) -> ("Microstep Size"=w263:dbl, "Device"=w262:string)
            n188 = call "Move.vi"("Units (0: microsteps)"=w279, "Movement Type (0: relative)"=w281, "Move Distance (0)"="GoTo X [mm]", "error in (no error)"=w269, "Device and Axis"=w262, "Microstep Size (0)"=w263, "VISA resource name"=w271) -> ("error out"=w280:errorcluster, "VISA resource name out"=w264:refnum<visa-resource-name>)  [unwired: 3 in]
            n189 = local write "ZaberError"(w280) -> ()
            n190 = call "Read Current Position.vi"("Device and Axis"=w262, "Microstep Size (0)"=w263, "VISA resource name"=w264) -> ()  [unwired: 6 in, 3 out]
          }
          event "GoToZ": Value Change {
            w293 = u16 2 items=["device units", "microns/s^2", "mm/s^2", "inches/s^2", "degrees/s^2"] ("Units (0: data)")
            w295 = u16 2 items=["device speed units", "microns per second", "millimeters per second", "inches per second", "degrees per second"] ("Units (0: device speed units)")
            w302 = u16 2 items=["microsteps", "microns", "millimeters", "inches", "degrees"] ("Units (0: microsteps)")
            w305 = u16 1 items=["relative", "absolute"] ("Movement Type (0: relative)")
            # "move to point command"
            n191 = event-data() -> ()  [unwired: 1 in, 6 out]
            n192 = local read "Assignment"() -> (w301:cluster{"Microstep Size":dbl, "Device":string}[])
            n193 = local read "ZaberError"() -> (w294:errorcluster)
            n194 = Index Array(array=w301, index=2) -> (element=w300:cluster{"Microstep Size":dbl, "Device":string})
            n195 = local read "Speed Z [mm/s]"() -> (w296:dbl)
            n196 = local read "Port"() -> (w297:refnum<visa-resource-name>)
            n197 = Unbundle(w300) -> ("Microstep Size"=w287:dbl, "Device"=w288:string)
            n198 = call "Set Speed.vi"("Units (0: data)"=w295, "New Speed"=w296, "error in (no error)"=w294, "Device and Axis"=w288, "Microstep Size (0)"=w287, "VISA resource name"=w297) -> ("error out"=w290:errorcluster, "VISA resource name out"=w292:refnum<visa-resource-name>)  [unwired: 4 in]
            n199 = local read "Acceleration [mm/s^2]"() -> (w286:dbl)
            n200 = call "Set Acceleration.vi"("Units (0: data)"=w293, "New Acceleration"=w286, "error in (no error)"=w290, "Device and Axis"=w288, "Microstep Size (0)"=w287, "VISA resource name"=w292) -> ("error out"=w289:errorcluster, "VISA resource name out"=w291:refnum<visa-resource-name>)  [unwired: 4 in]
            n201 = Unbundle(w300) -> ("Microstep Size"=w299:dbl, "Device"=w298:string)
            n202 = call "Move.vi"("Units (0: microsteps)"=w302, "Movement Type (0: relative)"=w305, "Move Distance (0)"="GoTo Z [mm]", "error in (no error)"=w289, "Device and Axis"=w298, "Microstep Size (0)"=w299, "VISA resource name"=w291) -> ("error out"=w304:errorcluster)  [unwired: 3 in, 1 out]
            n203 = local write "ZaberError"(w304) -> ()
          }
          event "StopMotion": Value Change {
            # "stop command"
            n204 = event-data() -> ()  [unwired: 1 in, 6 out]
            n205 = local read "Assignment"() -> (w312:cluster{"Microstep Size":dbl, "Device":string}[])
            n206 = local read "ZaberError"() -> (w310:errorcluster)
            n207 = local read "Port"() -> (w311:refnum<visa-resource-name>)
            n208 = for {
              tunnel: w312 -> [w316] mode=indexing
              shift-right: [w317] -> _
              shift-left: w311 -> [w320]
              shift-right: [w318] -> w309
              shift-left: w310 -> [w319]
              n209 = Unbundle(w316) -> ("Device"=w315:string)  [unwired: 1 out]
              n210 = call "Stop.vi"("error in (no error)"=w319, "Device and Axis"=w315, "VISA resource name"=w320) -> ("error out"=w318:errorcluster, "VISA resource name out"=w317:refnum<visa-resource-name>)  [unwired: 7 in]
            }
            n211 = local write "ZaberError"(w309) -> ()
          }
          event "Down": Value Change {
            n212 = event-data() -> ("NewVal"=w324:bool)  [unwired: 1 in, 5 out]
            n213 = local read "Assignment"() -> (w321:cluster{"Microstep Size":dbl, "Device":string}[])
            n214 = Index Array(array=w321, index=1) -> (element=w322:cluster{"Microstep Size":dbl, "Device":string})
            n215 = case shown="True" w324 {
              tunnel: w322 -> [_ w342]
              frame False {
                # "stop command"
                n216 = local read "Port"() -> (w329:refnum<visa-resource-name>)
                n217 = local read "ZaberError"() -> (w328:errorcluster)
                n218 = call "Stop.vi"("error in (no error)"=w328, "VISA resource name"=w329) -> ("error out"=w327:errorcluster)  [unwired: 8 in, 1 out]
                n219 = local write "ZaberError"(w327) -> ()
              }
              frame True {
                w341 = u16 2 items=["device units", "microns/s^2", "mm/s^2", "inches/s^2", "degrees/s^2"] ("Units (0: data)")
                w332 = u16 2 items=["device speed units", "microns per second", "millimeters per second", "inches per second", "degrees per second"] ("Units (0: device speed units)")
                # "move at specified velocity command"
                n220 = local read "Acceleration [mm/s^2]"() -> (w340:dbl)
                n221 = local read "ZaberError"() -> (w338:errorcluster)
                n222 = local read "Port"() -> (w339:refnum<visa-resource-name>)
                n223 = local read "XY Speed\n[mm/s]"() -> (w333:dbl)
                n224 = Unbundle(w342) -> ("Microstep Size"=w330:dbl, "Device"=w331:string)
                n225 = call "Set Acceleration.vi"("Units (0: data)"=w341, "New Acceleration"=w340, "error in (no error)"=w338, "Device and Axis"=w331, "Microstep Size (0)"=w330, "VISA resource name"=w339) -> ("error out"=w336:errorcluster, "VISA resource name out"=w337:refnum<visa-resource-name>)  [unwired: 4 in]
                n226 = call "Move at Velocity.vi"("Units (0: device speed units)"=w332, "Velocity"=w333, "error in (no error)"=w336, "Device and Axis"=w331, "Microstep Size (0)"=w330, "VISA resource name"=w337) -> ("error out"=w334:errorcluster, "VISA resource name out"=w335:refnum<visa-resource-name>)  [unwired: 4 in]
                n227 = while {
                  shift-right: [w348] -> _
                  shift-left: w335 -> [w351]
                  shift-right: [w349] -> w343
                  shift-left: w334 -> [w350]
                  tunnel: w342 -> [w344]
                  stop <- w354 stop-if-true
                  w353 = u16 2 items=["microsteps", "microns", "millimeters", "inches"] ("Units (0: microsteps)")
                  n228 = Wait (ms)(milliseconds to wait=u32 100) -> ()  [unwired: 1 out]
                  n229 = Unbundle(w344) -> ("Microstep Size"=w346:dbl, "Device"=w345:string)
                  n230 = call "Read Current Position.vi"("Units (0: microsteps)"=w353, "error in (no error)"=w350, "Device and Axis"=w345, "Microstep Size (0)"=w346, "VISA resource name"=w351) -> ("error out"=w349:errorcluster, "Position"=w352:dbl, "VISA resource name out"=w348:refnum<visa-resource-name>)  [unwired: 4 in]
                  n231 = Not(x="Down") -> (.not. x?=w354:bool)
                  n232 = local write "Y [mm]"(w352) -> ()
                }
                n233 = local write "ZaberError"(w343) -> ()
              }
            }
          }
          event "Closer": Value Change {
            n234 = event-data() -> ("NewVal"=w357:bool)  [unwired: 1 in, 5 out]
            n235 = local read "Assignment"() -> (w356:cluster{"Microstep Size":dbl, "Device":string}[])
            n236 = Index Array(array=w356, index=2) -> (element=w358:cluster{"Microstep Size":dbl, "Device":string})
            n237 = case shown="True" w357 {
              tunnel: w358 -> [_ w377]
              frame False {
                # "stop command"
                n238 = local read "Port"() -> (w364:refnum<visa-resource-name>)
                n239 = local read "ZaberError"() -> (w363:errorcluster)
                n240 = call "Stop.vi"("error in (no error)"=w363, "VISA resource name"=w364) -> ("error out"=w362:errorcluster)  [unwired: 8 in, 1 out]
                n241 = local write "ZaberError"(w362) -> ()
              }
              frame True {
                w375 = u16 2 items=["device units", "microns/s^2", "mm/s^2", "inches/s^2", "degrees/s^2"] ("Units (0: data)")
                w369 = u16 2 items=["device speed units", "microns per second", "millimeters per second", "inches per second", "degrees per second"] ("Units (0: device speed units)")
                # "move at specified velocity command"
                n242 = local read "Acceleration [mm/s^2]"() -> (w376:dbl)
                n243 = local read "ZaberError"() -> (w373:errorcluster)
                n244 = local read "Speed Z [mm/s]"() -> (w368:dbl)
                n245 = local read "Port"() -> (w374:refnum<visa-resource-name>)
                n246 = Unbundle(w377) -> ("Microstep Size"=w371:dbl, "Device"=w370:string)
                n247 = call "Set Acceleration.vi"("Units (0: data)"=w375, "New Acceleration"=w376, "error in (no error)"=w373, "Device and Axis"=w370, "Microstep Size (0)"=w371, "VISA resource name"=w374) -> ("error out"=w372:errorcluster, "VISA resource name out"=w366:refnum<visa-resource-name>)  [unwired: 4 in]
                n248 = call "Move at Velocity.vi"("Units (0: device speed units)"=w369, "Velocity"=w368, "error in (no error)"=w372, "Device and Axis"=w370, "Microstep Size (0)"=w371, "VISA resource name"=w366) -> ("error out"=w367:errorcluster, "VISA resource name out"=w365:refnum<visa-resource-name>)  [unwired: 4 in]
                n249 = while {
                  shift-right: [w384] -> _
                  shift-left: w365 -> [w387]
                  shift-right: [w385] -> w378
                  shift-left: w367 -> [w386]
                  tunnel: w377 -> [w379]
                  stop <- w389 stop-if-true
                  w388 = u16 2 items=["microsteps", "microns", "millimeters", "inches"] ("Units (0: microsteps)")
                  n250 = Wait (ms)(milliseconds to wait=u32 100) -> ()  [unwired: 1 out]
                  n251 = Unbundle(w379) -> ("Microstep Size"=w381:dbl, "Device"=w380:string)
                  n252 = call "Read Current Position.vi"("Units (0: microsteps)"=w388, "error in (no error)"=w386, "Device and Axis"=w380, "Microstep Size (0)"=w381, "VISA resource name"=w387) -> ("error out"=w385:errorcluster, "Position"=w383:dbl, "VISA resource name out"=w384:refnum<visa-resource-name>)  [unwired: 4 in]
                  n253 = Not(x="Closer") -> (.not. x?=w389:bool)
                  n254 = local write "Z [mm]"(w383) -> ()
                }
                n255 = local write "ZaberError"(w378) -> ()
              }
            }
          }
          event "Left": Value Change {
            n256 = event-data() -> ("NewVal"=w392:bool)  [unwired: 1 in, 5 out]
            n257 = local read "Assignment"() -> (w391:cluster{"Microstep Size":dbl, "Device":string}[])
            n258 = Index Array(array=w391, index=0) -> (element=w393:cluster{"Microstep Size":dbl, "Device":string})
            n259 = case shown="True" w392 {
              tunnel: w393 -> [_ w412]
              frame False {
                # "stop command"
                n260 = local read "Port"() -> (w399:refnum<visa-resource-name>)
                n261 = local read "ZaberError"() -> (w398:errorcluster)
                n262 = call "Stop.vi"("error in (no error)"=w398, "VISA resource name"=w399) -> ("error out"=w397:errorcluster)  [unwired: 8 in, 1 out]
                n263 = local write "ZaberError"(w397) -> ()
              }
              frame True {
                w411 = u16 2 items=["device units", "microns/s^2", "mm/s^2", "inches/s^2", "degrees/s^2"] ("Units (0: data)")
                w401 = u16 2 items=["device speed units", "microns per second", "millimeters per second", "inches per second", "degrees per second"] ("Units (0: device speed units)")
                # "move at specified velocity command"
                n264 = local read "ZaberError"() -> (w408:errorcluster)
                n265 = local read "XY Speed\n[mm/s]"() -> (w413:dbl)
                n266 = local read "Port"() -> (w409:refnum<visa-resource-name>)
                n267 = Negate(x=w413) -> (-x=w400:dbl)
                n268 = local read "Acceleration [mm/s^2]"() -> (w410:dbl)
                n269 = Unbundle(w412) -> ("Microstep Size"=w403:dbl, "Device"=w402:string)
                n270 = call "Set Acceleration.vi"("Units (0: data)"=w411, "New Acceleration"=w410, "error in (no error)"=w408, "Device and Axis"=w402, "Microstep Size (0)"=w403, "VISA resource name"=w409) -> ("error out"=w406:errorcluster, "VISA resource name out"=w407:refnum<visa-resource-name>)  [unwired: 4 in]
                n271 = call "Move at Velocity.vi"("Units (0: device speed units)"=w401, "Velocity"=w400, "error in (no error)"=w406, "Device and Axis"=w402, "Microstep Size (0)"=w403, "VISA resource name"=w407) -> ("error out"=w404:errorcluster, "VISA resource name out"=w405:refnum<visa-resource-name>)  [unwired: 4 in]
                n272 = while {
                  shift-right: [w420] -> _
                  shift-left: w405 -> [w423]
                  shift-right: [w421] -> w414
                  shift-left: w404 -> [w422]
                  tunnel: w412 -> [w417]
                  stop <- w425 stop-if-true
                  w424 = u16 2 items=["microsteps", "microns", "millimeters", "inches"] ("Units (0: microsteps)")
                  n273 = Unbundle(w417) -> ("Microstep Size"=w416:dbl, "Device"=w415:string)
                  n274 = Wait (ms)(milliseconds to wait=u32 100) -> ()  [unwired: 1 out]
                  n275 = call "Read Current Position.vi"("Units (0: microsteps)"=w424, "error in (no error)"=w422, "Device and Axis"=w415, "Microstep Size (0)"=w416, "VISA resource name"=w423) -> ("error out"=w421:errorcluster, "Position"=w419:dbl, "VISA resource name out"=w420:refnum<visa-resource-name>)  [unwired: 4 in]
                  n276 = Not(x="Left") -> (.not. x?=w425:bool)
                  n277 = local write "X [mm]"(w419) -> ()
                }
                n278 = local write "ZaberError"(w414) -> ()
              }
            }
          }
          event "Right": Value Change {
            n279 = event-data() -> ("NewVal"=w428:bool)  [unwired: 1 in, 5 out]
            n280 = local read "Assignment"() -> (w427:cluster{"Microstep Size":dbl, "Device":string}[])
            n281 = Index Array(array=w427, index=0) -> (element=w429:cluster{"Microstep Size":dbl, "Device":string})
            n282 = case shown="True" w428 {
              tunnel: w429 -> [_ w448]
              frame False {
                # "stop command"
                n283 = local read "Port"() -> (w435:refnum<visa-resource-name>)
                n284 = local read "ZaberError"() -> (w434:errorcluster)
                n285 = call "Stop.vi"("error in (no error)"=w434, "VISA resource name"=w435) -> ("error out"=w433:errorcluster)  [unwired: 8 in, 1 out]
                n286 = local write "ZaberError"(w433) -> ()
              }
              frame True {
                w447 = u16 2 items=["device units", "microns/s^2", "mm/s^2", "inches/s^2", "degrees/s^2"] ("Units (0: data)")
                w437 = u16 2 items=["device speed units", "microns per second", "millimeters per second", "inches per second", "degrees per second"] ("Units (0: device speed units)")
                # "move at specified velocity command"
                n287 = local read "Acceleration [mm/s^2]"() -> (w446:dbl)
                n288 = local read "ZaberError"() -> (w445:errorcluster)
                n289 = local read "XY Speed\n[mm/s]"() -> (w436:dbl)
                n290 = local read "Port"() -> (w444:refnum<visa-resource-name>)
                n291 = Unbundle(w448) -> ("Microstep Size"=w439:dbl, "Device"=w438:string)
                n292 = call "Set Acceleration.vi"("Units (0: data)"=w447, "New Acceleration"=w446, "error in (no error)"=w445, "Device and Axis"=w438, "Microstep Size (0)"=w439, "VISA resource name"=w444) -> ("error out"=w443:errorcluster, "VISA resource name out"=w442:refnum<visa-resource-name>)  [unwired: 4 in]
                n293 = call "Move at Velocity.vi"("Units (0: device speed units)"=w437, "Velocity"=w436, "error in (no error)"=w443, "Device and Axis"=w438, "Microstep Size (0)"=w439, "VISA resource name"=w442) -> ("error out"=w440:errorcluster, "VISA resource name out"=w441:refnum<visa-resource-name>)  [unwired: 4 in]
                n294 = while {
                  shift-right: [w455] -> _
                  shift-left: w441 -> [w458]
                  shift-right: [w456] -> w449
                  shift-left: w440 -> [w457]
                  tunnel: w448 -> [w450]
                  stop <- w460 stop-if-true
                  w459 = u16 2 items=["microsteps", "microns", "millimeters", "inches"] ("Units (0: microsteps)")
                  n295 = Wait (ms)(milliseconds to wait=u32 100) -> ()  [unwired: 1 out]
                  n296 = Unbundle(w450) -> ("Microstep Size"=w452:dbl, "Device"=w451:string)
                  n297 = call "Read Current Position.vi"("Units (0: microsteps)"=w459, "error in (no error)"=w457, "Device and Axis"=w451, "Microstep Size (0)"=w452, "VISA resource name"=w458) -> ("error out"=w456:errorcluster, "Position"=w454:dbl, "VISA resource name out"=w455:refnum<visa-resource-name>)  [unwired: 4 in]
                  n298 = Not(x="Right") -> (.not. x?=w460:bool)
                  n299 = local write "X [mm]"(w454) -> ()
                }
                n300 = local write "ZaberError"(w449) -> ()
              }
            }
          }
          event "Away": Value Change {
            n301 = event-data() -> ("NewVal"=w463:bool)  [unwired: 1 in, 5 out]
            n302 = local read "Assignment"() -> (w462:cluster{"Microstep Size":dbl, "Device":string}[])
            n303 = Index Array(array=w462, index=2) -> (element=w464:cluster{"Microstep Size":dbl, "Device":string})
            n304 = case shown="True" w463 {
              tunnel: w464 -> [_ w483]
              frame False {
                # "stop command"
                n305 = local read "Port"() -> (w470:refnum<visa-resource-name>)
                n306 = local read "ZaberError"() -> (w469:errorcluster)
                n307 = call "Stop.vi"("error in (no error)"=w469, "VISA resource name"=w470) -> ("error out"=w468:errorcluster)  [unwired: 8 in, 1 out]
                n308 = local write "ZaberError"(w468) -> ()
              }
              frame True {
                w482 = u16 2 items=["device units", "microns/s^2", "mm/s^2", "inches/s^2", "degrees/s^2"] ("Units (0: data)")
                w476 = u16 2 items=["device speed units", "microns per second", "millimeters per second", "inches per second", "degrees per second"] ("Units (0: device speed units)")
                # "move at specified velocity command"
                n309 = local read "Acceleration [mm/s^2]"() -> (w481:dbl)
                n310 = local read "Speed Z [mm/s]"() -> (w484:dbl)
                n311 = local read "Port"() -> (w479:refnum<visa-resource-name>)
                n312 = local read "ZaberError"() -> (w480:errorcluster)
                n313 = Negate(x=w484) -> (-x=w475:dbl)
                n314 = Unbundle(w483) -> ("Microstep Size"=w478:dbl, "Device"=w477:string)
                n315 = call "Set Acceleration.vi"("Units (0: data)"=w482, "New Acceleration"=w481, "error in (no error)"=w480, "Device and Axis"=w477, "Microstep Size (0)"=w478, "VISA resource name"=w479) -> ("error out"=w473:errorcluster, "VISA resource name out"=w474:refnum<visa-resource-name>)  [unwired: 4 in]
                n316 = call "Move at Velocity.vi"("Units (0: device speed units)"=w476, "Velocity"=w475, "error in (no error)"=w473, "Device and Axis"=w477, "Microstep Size (0)"=w478, "VISA resource name"=w474) -> ("error out"=w472:errorcluster, "VISA resource name out"=w471:refnum<visa-resource-name>)  [unwired: 4 in]
                n317 = while {
                  shift-right: [w491] -> _
                  shift-left: w471 -> [w494]
                  shift-right: [w492] -> w485
                  shift-left: w472 -> [w493]
                  tunnel: w483 -> [w488]
                  stop <- w496 stop-if-true
                  w495 = u16 2 items=["microsteps", "microns", "millimeters", "inches"] ("Units (0: microsteps)")
                  n318 = Unbundle(w488) -> ("Microstep Size"=w487:dbl, "Device"=w486:string)
                  n319 = Wait (ms)(milliseconds to wait=u32 100) -> ()  [unwired: 1 out]
                  n320 = call "Read Current Position.vi"("Units (0: microsteps)"=w495, "error in (no error)"=w493, "Device and Axis"=w486, "Microstep Size (0)"=w487, "VISA resource name"=w494) -> ("error out"=w492:errorcluster, "Position"=w490:dbl, "VISA resource name out"=w491:refnum<visa-resource-name>)  [unwired: 4 in]
                  n321 = Not(x="Away") -> (.not. x?=w496:bool)
                  n322 = local write "Z [mm]"(w490) -> ()
                }
                n323 = local write "ZaberError"(w485) -> ()
              }
            }
          }
          event "Reduced Speed": Value Change {
            n324 = event-data() -> ("NewVal"=w512:bool)  [unwired: 1 in, 5 out]
            n325 = case shown="False" w512 {
              tunnel: [1.0 ("Minimum") 0.1 ("Minimum")] -> w509
              tunnel: [75.0 ("Minimum") 7.5 ("Minimum")] -> w508
              tunnel: [1.0 ("Minimum") 0.1 ("Minimum")] -> w507
              tunnel: [0.5 ("Minimum") 0.05 ("Minimum")] -> w500
              tunnel: [10.0 ("Minimum") 1.0 ("Minimum")] -> w499
              tunnel: [0.5 ("Minimum") 0.05 ("Minimum")] -> w498
              frame False {
                # "full speed"
              }
              frame True {
                # "reduced speed"
              }
            }
            n326 = property on="Speed Z [mm/s]" class="Slide (strict)"() -> ("Data Range"=w502:T9, "Scale.Range"=w501:T10)  [unwired: 2 in, 2 out]
            n327 = property on="XY Speed\n[mm/s]" class="Slide (strict)"() -> ("Data Range"=w514:T9, "Scale.Range"=w506:T10)  [unwired: 2 in, 2 out]
            n328 = Bundle By Name(cluster=w514, "Minimum"=w509, "Maximum"=w508, "Increment"=w507) -> (w513:T9)
            n329 = Bundle By Name(cluster=w506, "Minimum"=w509, "Maximum"=w508, "Increment"=w507) -> (w505:T10)
            n330 = Bundle By Name(cluster=w502, "Minimum"=w500, "Maximum"=w499, "Increment"=w498) -> (w504:T9)
            n331 = Bundle By Name(cluster=w501, "Minimum"=w500, "Maximum"=w499, "Increment"=w498) -> (w503:T10)
            n332 = property on="XY Speed\n[mm/s]" class="Slide (strict)"("Data Range"=w513, "Scale.Range"=w505) -> ()  [unwired: 2 in, 2 out]
            n333 = property on="Speed Z [mm/s]" class="Slide (strict)"("Data Range"=w504, "Scale.Range"=w503) -> ()  [unwired: 2 in, 2 out]
          }
          event Panel Close? {
            n334 = event-data() -> ()  [unwired: 1 in, 4 out]
            n335 = local read "DANTE configured"() -> (w528:bool)
            n336 = case shown="True" w528 {
              tunnel: [fast_scanner."Close" ("Enum") fast_scanner."IDLE" ("Enum")] -> w527
              frame False {
              }
              frame True {
                n337 = One Button Dialog(message="Close DANTE first") -> ()  [unwired: 1 in, 1 out]
              }
            }
            n338 = event-data("Discard?"=TRUE) -> ()  [unwired: 1 in, 1 out]
          }
          event "MEASUREMENT_Start": Value Change {
            n339 = event-data() -> ()  [unwired: 1 in, 5 out]
          }
          event "SpectraPlot": Mouse Up {
            (unwired) FALSE
            n340 = event-data() -> ()  [unwired: 1 in, 8 out]
            n341 = control-ref of="SpectraPlot"() -> (w541:refnum<vi>)
            n342 = property class="WFGraph (strict)"(reference=w541, "Active Cursor"=u32 1, "Active Cursor"=u32 2) -> ("Cursor.Cursor X"=w538:dbl, "Cursor.Cursor X"=w539:dbl)  [unwired: 1 in, 2 out]
            n343 = Less?(x=w538, y=w539) -> (x < y?=w540:bool)
            n344 = case shown="False" w540 {
              tunnel: w538 -> [w546 w549]
              tunnel: w539 -> [w547 w548]
              tunnel: [w547 w549] -> w542
              tunnel: [w546 w548] -> w543
              frame False {
              }
              frame True {
              }
            }
            "ROI Begin" <- w542
            "ROI End" <- w543
          }
          event "APPEARANCE_CursorVis": Value Change {
            n345 = event-data() -> ("NewVal"=w551:bool)  [unwired: 1 in]
            n346 = property on="SpectraPlot" class="WFGraph (strict)"("Cursor Palette Vis"=w551, "Active Cursor"=u32 0, "Cursor.Visible"=w551) -> ()  [unwired: 2 in, 2 out]
          }
          event "APPEARANCE_Log/Lin": Value Change {
            n347 = event-data() -> ("NewVal"=w556:bool)  [unwired: 1 in]
            n348 = Boolean To (0,1)(Boolean=w556) -> (0, 1=w555:i16)
            n349 = property on="SpectraPlot" class="WFGraph (strict)"("YScale.Mapping Mode"=w555) -> ()  [unwired: 2 in, 2 out]
          }
        }
      }
      frame "Acquire" {
        # "if not mapping plot last spectra on spectra plot"
        n350 = local read "identifier out"() -> (w561:string)
        n351 = call "DANTE acquire single.vi"("Acquisition time [s]"="Preset Time [s]", "identifier out"=w561) -> ("stats out"=→"stats out":T4, "single spectrum"=→"SpectraPlot":dbl[])  [unwired: 8 in]
      }
      frame "PrepareMap" {
        n352 = local read "X start [mm]"() -> (w577:dbl)
        n353 = local read "Y start [mm]"() -> (w582:dbl)
        n354 = local read "step Y [mm]"() -> (w579:dbl)
        n355 = local read "X [mm]"() -> (w576:dbl)
        n356 = local read "Y [mm]"() -> (w581:dbl)
        n357 = local read "X end [mm]"() -> (w572:dbl)
        n358 = local read "X [mm]"() -> (w571:dbl)
        n359 = local read "Y steps"() -> (w569:i32)
        "total line #" <- w569
        n360 = Add(x=w577, y=w576) -> (x+y=→"X start position":dbl)
        n361 = Add(x=w572, y=w571) -> (x+y=→"X end position":dbl)
        n362 = Add(x=w581, y=w582) -> (x+y=w580:dbl)
        n363 = for {
          N: w569 -> [_]
          tunnel: w580 -> [w590]
          tunnel: w579 -> [w591]
          tunnel: [w588] -> w578 mode=indexing
          i -> [w592]
          n364 = Multiply(x=w591, y=w592) -> (x*y=w589:dbl)
          n365 = Add(x=w590, y=w589) -> (x+y=w588:dbl)
        }
        "Y positions array" <- w578
        n366 = local read "X steps"() -> (w566:i32)
        n367 = local read "Y steps"() -> (w565:i32)
        n368 = Initialize Array(u32 0 ("element"), w566, w565) -> (→"ROI map":u32[][])
        n369 = for {
          N: w569 -> [_]
          tunnel: [w585] -> w568 mode=indexing
          n370 = Initialize Array(0.0 ("element"), 4 ("dimension size")) -> (w585:dbl[])
        }
        "scan timing [ms]" <- w568
        "scan mode" <- TRUE ("scan mode")
        "Line #" <- 1 ("Line #")
      }
      frame "MoveToStartPoint" {
        n371 = stacked-sequence {
          frame #0 {
            w600 = u16 2 items=["device units", "microns/s^2", "mm/s^2", "inches/s^2", "degrees/s^2"] ("Units (0: data)")
            w608 = u16 2 items=["device speed units", "microns per second", "millimeters per second", "inches per second", "degrees per second"] ("Units (0: device speed units)")
            w614 = u16 2 items=["microsteps", "microns", "millimeters", "inches", "degrees"] ("Units (0: microsteps)")
            w616 = u16 1 items=["relative", "absolute"] ("Movement Type (0: relative)")
            n372 = local read "Y positions array"() -> (w599:dbl[])
            n373 = local read "Line #"() -> (w598:i32)
            n374 = local read "Assignment"() -> (w613:cluster{"Microstep Size":dbl, "Device":string}[])
            n375 = Index Array(array=w599, index=w598) -> (element=w597:dbl)
            n376 = Index Array(array=w613, index=1) -> (element=w610:cluster{"Microstep Size":dbl, "Device":string})
            n377 = local read "Port"() -> (w607:refnum<visa-resource-name>)
            n378 = local read "ZaberError"() -> (w609:errorcluster)
            n379 = local read "X velocity [mm/s]"() -> (w595:dbl)
            n380 = Unbundle(w610) -> ("Microstep Size"=w606:dbl, "Device"=w605:string)
            n381 = call "Set Speed.vi"("Units (0: data)"=w608, "New Speed"=w595, "error in (no error)"=w609, "Device and Axis"=w605, "Microstep Size (0)"=w606, "VISA resource name"=w607) -> ("error out"=w604:errorcluster, "VISA resource name out"=w602:refnum<visa-resource-name>)  [unwired: 4 in]
            n382 = local read "X accel"() -> (w596:dbl)
            n383 = call "Set Acceleration.vi"("Units (0: data)"=w600, "New Acceleration"=w596, "error in (no error)"=w604, "Device and Axis"=w605, "Microstep Size (0)"=w606, "VISA resource name"=w602) -> ("error out"=w603:errorcluster, "VISA resource name out"=w601:refnum<visa-resource-name>)  [unwired: 4 in]
            n384 = Unbundle(w610) -> ("Microstep Size"=w612:dbl, "Device"=w611:string)
            n385 = call "Move.vi"("Units (0: microsteps)"=w614, "Movement Type (0: relative)"=w616, "Move Distance (0)"=w597, "error in (no error)"=w603, "Device and Axis"=w611, "Microstep Size (0)"=w612, "VISA resource name"=w601) -> ("error out"=w615:errorcluster)  [unwired: 3 in, 1 out]
            n386 = local write "ZaberError"(w615) -> ()
          }
          frame #1 {
            w623 = u16 2 items=["device units", "microns/s^2", "mm/s^2", "inches/s^2", "degrees/s^2"] ("Units (0: data)")
            w634 = u16 2 items=["device speed units", "microns per second", "millimeters per second", "inches per second", "degrees per second"] ("Units (0: device speed units)")
            w637 = u16 2 items=["microsteps", "microns", "millimeters", "inches", "degrees"] ("Units (0: microsteps)")
            w639 = u16 1 items=["relative", "absolute"] ("Movement Type (0: relative)")
            # "move to point command"
            n387 = local read "Assignment"() -> (w633:cluster{"Microstep Size":dbl, "Device":string}[])
            n388 = local read "Port"() -> (w635:refnum<visa-resource-name>)
            n389 = Index Array(array=w633, index=0) -> (element=w630:cluster{"Microstep Size":dbl, "Device":string})
            n390 = local read "ZaberError"() -> (w636:errorcluster)
            n391 = local read "X velocity [mm/s]"() -> (w618:dbl)
            n392 = Unbundle(w630) -> ("Microstep Size"=w625:dbl, "Device"=w624:string)
            n393 = call "Set Speed.vi"("Units (0: data)"=w634, "New Speed"=w618, "error in (no error)"=w636, "Device and Axis"=w624, "Microstep Size (0)"=w625, "VISA resource name"=w635) -> ("error out"=w627:errorcluster, "VISA resource name out"=w629:refnum<visa-resource-name>)  [unwired: 4 in]
            n394 = local read "X start position"() -> (w622:dbl)
            n395 = local read "Acc dist [mm]"() -> (w621:dbl)
            n396 = local read "X accel"() -> (w619:dbl)
            n397 = call "Set Acceleration.vi"("Units (0: data)"=w623, "New Acceleration"=w619, "error in (no error)"=w627, "Device and Axis"=w624, "Microstep Size (0)"=w625, "VISA resource name"=w629) -> ("error out"=w626:errorcluster, "VISA resource name out"=w628:refnum<visa-resource-name>)  [unwired: 4 in]
            n398 = Subtract(x=w622, y=w621) -> (x-y=w620:dbl)
            n399 = Unbundle(w630) -> ("Microstep Size"=w632:dbl, "Device"=w631:string)
            n400 = call "Move.vi"("Units (0: microsteps)"=w637, "Movement Type (0: relative)"=w639, "Move Distance (0)"=w620, "error in (no error)"=w626, "Device and Axis"=w631, "Microstep Size (0)"=w632, "VISA resource name"=w628) -> ("error out"=w638:errorcluster)  [unwired: 3 in, 1 out]
            n401 = local write "ZaberError"(w638) -> ()
          }
          frame #2 {
            n402 = disable-structure shown="Disabled" {
              frame Disabled {
                # "wait till movement is completed"
                n403 = while {
                  stop <- w656 stop-if-true
                  w665 = u16 2 items=["microsteps", "microns", "millimeters", "inches"] ("Units (0: microsteps)")
                  # "Y"
                  # "X"
                  n404 = local read "Assignment"() -> (w666:cluster{"Microstep Size":dbl, "Device":string}[])
                  n405 = local read "ZaberError"() -> (w660:errorcluster)
                  n406 = local read "Port"() -> (w659:refnum<visa-resource-name>)
                  n407 = local read "X start position"() -> (w646:dbl)
                  n408 = local read "Acc dist [mm]"() -> (w645:dbl)
                  n409 = Index Array(array=w666, index=0) -> (element=w667:cluster{"Microstep Size":dbl, "Device":string})
                  n410 = Index Array(array=w666, index=1) -> (element=w668:cluster{"Microstep Size":dbl, "Device":string})
                  n411 = Subtract(x=w646, y=w645) -> (x-y=w644:dbl)
                  n412 = Unbundle(w667) -> ("Microstep Size"=w651:dbl, "Device"=w652:string)
                  n413 = call "Read Current Position.vi"("Units (0: microsteps)"=w665, "error in (no error)"=w660, "Device and Axis"=w652, "Microstep Size (0)"=w651, "VISA resource name"=w659) -> ("error out"=w661:errorcluster, "Position"=w650:dbl, "VISA resource name out"=w662:refnum<visa-resource-name>)  [unwired: 4 in]
                  n414 = local read "Y positions array"() -> (w642:dbl[])
                  n415 = call "ChkOnTarget.vi"("Prec"="Precision [mm]", "TargetPos"=w644, "CurrPos"=w650) -> ("In Range?"=w657:bool)
                  n416 = local read "Line #"() -> (w643:i32)
                  n417 = Unbundle(w668) -> ("Microstep Size"=w648:dbl, "Device"=w649:string)
                  n418 = Index Array(array=w642, index=w643) -> (element=w641:dbl)
                  n419 = call "Read Current Position.vi"("Units (0: microsteps)"=w665, "error in (no error)"=w661, "Device and Axis"=w649, "Microstep Size (0)"=w648, "VISA resource name"=w662) -> ("error out"=w654:errorcluster, "Position"=w647:dbl, "VISA resource name out"=w653:refnum<visa-resource-name>)  [unwired: 4 in]
                  n420 = call "ChkOnTarget.vi"("Prec"="Precision [mm]", "TargetPos"=w641, "CurrPos"=w647) -> ("In Range?"=w658:bool)
                  n421 = local write "Port"(w653) -> ()
                  n422 = local write "ZaberError"(w654) -> ()
                  n423 = Compound Arithmetic op=AND(w658, w657) -> (w656:bool)
                }
              }
              frame Enabled {
              }
            }
          }
          frame #3 {
            # "wait till movement is completed"
            n424 = local read "Assignment"() -> (w671:cluster{"Microstep Size":dbl, "Device":string}[])
            n425 = local read "ZaberError"() -> (w674:errorcluster)
            n426 = local read "Port"() -> (w675:refnum<visa-resource-name>)
            n427 = Index Array(array=w671, index=0) -> (element=w672:cluster{"Microstep Size":dbl, "Device":string})
            n428 = Index Array(array=w671, index=1) -> (element=w673:cluster{"Microstep Size":dbl, "Device":string})
            n429 = Unbundle(w672) -> ("Device"=w676:string)  [unwired: 1 out]
            n430 = call "Poll Until Idle.vi"("error in (no error)"=w674, "Device and Axis"=w676, "VISA resource name"=w675) -> ("error out"=w678:errorcluster, "VISA resource name out"=w681:refnum<visa-resource-name>)  [unwired: 7 in]
            n431 = Unbundle(w673) -> ("Device"=w677:string)  [unwired: 1 out]
            n432 = call "Poll Until Idle.vi"("error in (no error)"=w678, "Device and Axis"=w677, "VISA resource name"=w681) -> ("error out"=w679:errorcluster, "VISA resource name out"=w680:refnum<visa-resource-name>)  [unwired: 7 in]
            n433 = local write "Port"(w680) -> ()
            n434 = local write "ZaberError"(w679) -> ()
          }
        }
      }
      frame "AcquireLine" {
        # "stats"
        # "spectra"
        # "acceleration"
        # "waiting till movement completed"
        # "acquisition command"
        # "sending movement command"
        n435 = stacked-sequence {
          seq-local: [w685 _ _ _ _ _ _ _ _ _ _ _] -> [_ _ w710 _ _ _ _ _ _ _ _ _]
          seq-local: [_ _ w711 _ _ _ _ _ _ _ _ _] -> [_ _ _ _ w718 _ _ _ _ _ _ _]
          seq-local: [_ _ _ _ w719 _ _ _ _ _ _ _] -> [_ _ _ _ _ _ w728 _ _ _ _ _]
          seq-local: [_ _ w709 _ _ _ _ _ _ _ _ _] -> [_ _ _ _ _ _ _ _ _ _ _ w767]
          seq-local: [_ _ _ _ _ _ w727 _ _ _ _ _] -> [_ _ _ _ _ _ _ _ _ _ _ w765]
          seq-local: [_ _ _ _ _ _ w726 _ _ _ _ _] -> [_ _ _ _ _ _ _ _ w737 _ _ _]
          seq-local: [_ _ _ _ _ _ _ _ w736 _ _ _] -> [_ _ _ _ _ _ _ _ _ _ _ w764]
          seq-local: [_ _ _ _ w717 _ _ _ _ _ _ _] -> [_ _ _ _ _ _ _ _ _ _ _ w766]
          seq-local: [_ _ _ _ _ w721 _ _ _ _ _ _] -> [_ _ _ _ _ _ _ _ _ w746 w754 _]
          seq-local: [_ _ _ _ _ w720 _ _ _ _ _ _] -> [_ _ _ _ _ _ _ _ _ _ w751 _]
          tunnel: [_ _ _ _ _ _ _ _ _ _ w750 _] -> _
          tunnel: w682 -> [_ _ _ _ _ _ _ _ _ _ w750 _]
          frame #0 {
            n436 = Tick Count (ms)() -> (millisecond timer value=w685:u32)
          }
          frame #1 {
            w708 = u16 2 items=["device units", "microns/s^2", "mm/s^2", "inches/s^2", "degrees/s^2"] ("Units (0: data)")
            w697 = u16 2 items=["device speed units", "microns per second", "millimeters per second", "inches per second", "degrees per second"] ("Units (0: device speed units)")
            w694 = u16 2 items=["microsteps", "microns", "millimeters", "inches", "degrees"] ("Units (0: microsteps)")
            w692 = u16 1 items=["relative", "absolute"] ("Movement Type (0: relative)")
            n437 = local read "Assignment"() -> (w698:cluster{"Microstep Size":dbl, "Device":string}[])
            n438 = local read "Port"() -> (w696:refnum<visa-resource-name>)
            n439 = Index Array(array=w698, index=0) -> (element=w701:cluster{"Microstep Size":dbl, "Device":string})
            n440 = local read "ZaberError"() -> (w695:errorcluster)
            n441 = local read "X scan velocity [mm/s]"() -> (w690:dbl)
            n442 = local read "X accel"() -> (w689:dbl)
            n443 = Unbundle(w701) -> ("Microstep Size"=w706:dbl, "Device"=w707:string)
            n444 = call "Set Speed.vi"("Units (0: data)"=w697, "New Speed"=w690, "error in (no error)"=w695, "Device and Axis"=w707, "Microstep Size (0)"=w706, "VISA resource name"=w696) -> ("error out"=w704:errorcluster, "VISA resource name out"=w702:refnum<visa-resource-name>)  [unwired: 4 in]
            n445 = local read "Acc dist [mm]"() -> (w686:dbl)
            n446 = local read "X end position"() -> (w687:dbl)
            n447 = call "Set Acceleration.vi"("Units (0: data)"=w708, "New Acceleration"=w689, "error in (no error)"=w704, "Device and Axis"=w707, "Microstep Size (0)"=w706, "VISA resource name"=w702) -> ("error out"=w705:errorcluster, "VISA resource name out"=w703:refnum<visa-resource-name>)  [unwired: 4 in]
            n448 = Add(x=w687, y=w686) -> (x+y=w688:dbl)
            n449 = Unbundle(w701) -> ("Microstep Size"=w699:dbl, "Device"=w700:string)
            n450 = call "Move.vi"("Units (0: microsteps)"=w694, "Movement Type (0: relative)"=w692, "Move Distance (0)"=w688, "error in (no error)"=w705, "Device and Axis"=w700, "Microstep Size (0)"=w699, "VISA resource name"=w703) -> ("error out"=w693:errorcluster)  [unwired: 3 in, 1 out]
            n451 = local write "ZaberError"(w693) -> ()
          }
          frame #2 {
            n452 = Tick Count (ms)() -> (millisecond timer value=w711:u32)
            n453 = Subtract(x=w711, y=w710) -> (x-y=w709:u32)
          }
          frame #3 {
            n454 = local read "Acc time [s]"() -> (w714:dbl)
            n455 = Multiply(x=1000.0 ("y"), y=w714) -> (x*y=w713:dbl)
            n456 = Add(x="AcqStartDelay", y=w713) -> (x+y=w712:dbl)
            n457 = Wait (ms)(milliseconds to wait=w712) -> ()  [unwired: 1 out]
          }
          frame #4 {
            n458 = Tick Count (ms)() -> (millisecond timer value=w719:u32)
            n459 = Subtract(x=w719, y=w718) -> (x-y=w717:u32)
          }
          frame #5 {
            # "acquisition command + waiting till acquisition is done (subVI is suppose to stop after finish)"
            n460 = local read "X steps"() -> (w723:i32)
            n461 = local read "identifier out"() -> (w725:string)
            n462 = call "DANTE acquire multiple.vi"("Number of boards in chain"=u8 1, "Map points"=w723, "Time per spectrum [ms]"="PresetVal", "identifier out"=w725) -> ("spectra"=w721:u16[][], "adv stats"=w720:u64[][])  [unwired: 6 in]
          }
          frame #6 {
            n463 = Tick Count (ms)() -> (millisecond timer value=w726:u32)
            n464 = Subtract(x=w726, y=w728) -> (x-y=w727:u32)
          }
          frame #7 {
            # "waiting till movement is completed - decelleration"
            n465 = local read "Assignment"() -> (w733:cluster{"Microstep Size":dbl, "Device":string}[])
            n466 = Index Array(array=w733, index=0) -> (element=w734:cluster{"Microstep Size":dbl, "Device":string})
            n467 = local read "ZaberError"() -> (w730:errorcluster)
            n468 = local read "Port"() -> (w735:refnum<visa-resource-name>)
            n469 = Unbundle(w734) -> ("Device"=w731:string)  [unwired: 1 out]
            n470 = call "Poll Until Idle.vi"("error in (no error)"=w730, "Device and Axis"=w731, "VISA resource name"=w735) -> ("error out"=w729:errorcluster)  [unwired: 7 in, 1 out]
            n471 = local write "ZaberError"(w729) -> ()
          }
          frame #8 {
            n472 = Tick Count (ms)() -> (millisecond timer value=w738:u32)
            n473 = Subtract(x=w738, y=w737) -> (x-y=w736:u32)
          }
          frame #9 {
            # "saving data"
            n474 = local read "ROI End"() -> (w741:u32)
            n475 = local read "ROI Begin"() -> (w742:u32)
            n476 = call "Extract LineData.vi"("ROI End"=w741, "Input Data"=w746, "ROI Beg"=w742) -> ("ROI Data"=w743:u32[], "Sum spectra"=→"Sum spectra":u32[])  [unwired: 1 out]
            n477 = local read "ROI map"() -> (w744:u32[][])
            n478 = local read "Line #"() -> (w740:i32)
            n479 = Replace Array Subset(array=w744, new element=w743, index (col)=w740) -> (w739:u32[][])  [unwired: 1 in]
            n480 = local write "ROI map"(w739) -> ()
            "Spectra" <- w746
          }
          frame #10 {
            w747 = ";"
            n481 = local read "Line #"() -> (w759:i32)
            n482 = Number To Decimal String(number=w759, width (-)=i16 1) -> (decimal integer string=w752:string)
            n483 = Concatenate Strings(w752, "_spectr.csv" ("string")) -> (w756:string)
            n484 = Concatenate Strings(w752, "_stat.csv" ("string")) -> (w749:string)
            n485 = Build Path(base path=w750, name or relative path=w756) -> (appended path=w755:path)
            n486 = Build Path(base path=w750, name or relative path=w749) -> (appended path=w748:path)
            n487 = call-poly <vilib>:"Write Delimited Spreadsheet.vi"("file path (dialog if empty)"=w755, "2D data"=w754, "delimiter (\\t)"=w747) -> ()  [unwired: 11 in, 2 out]
            n488 = call-poly <vilib>:"Write Delimited Spreadsheet.vi"("file path (dialog if empty)"=w748, "2D data"=w751, "delimiter (\\t)"=w747) -> ()  [unwired: 11 in, 2 out]
          }
          frame #11 {
            n489 = local read "total line #"() -> (w768:i32)
            n490 = local read "Line #"() -> (w761:i32)
            n491 = local read "scan timing [ms]"() -> (w762:dbl[][])
            n492 = Equal?(x=w768, y=w761) -> (x = y?=w769:bool)
            n493 = case shown="False" w769 {
              frame False {
                n494 = local read "Line #"() -> (w770:i32)
                n495 = Increment(x=w770) -> (x+1=w771:i32)
                n496 = local write "Line #"(w771) -> ()
              }
              frame True {
                n497 = local write "scan mode"(FALSE ("scan mode")) -> ()
              }
            }
            n498 = Build Array(w767, w766, w765, w764) -> (w763:u32[])
            n499 = Insert Into Array(array=w762, index (row)=w761, new element=w763) -> (w760:dbl[][])  [unwired: 1 in]
            n500 = local write "scan timing [ms]"(w760) -> ()
          }
        }
      }
      frame "Close" {
        n501 = local read "ZaberError"() -> (w776:errorcluster)
        n502 = local read "Port"() -> (w775:refnum<visa-resource-name>)
        n503 = call "Close.vi"("error in (no error)"=w776, "VISA resource name"=w775) -> ("error out"=→"ZaberError":errorcluster)  [unwired: 9 in]
      }
    }
    n504 = Reciprocal(x=w22) -> (1/x=→"Loop Speed [1/s]":dbl)
    n505 = Wait Until Next ms Multiple(millisecond multiple=u32 40) -> ()  [unwired: 1 out]
    "Enum" <- w8
  }
